vi "HyMPaCt Control Software.vi"() -> ()   [LabVIEW 2017]
doc: "This is the vi discription of the Top Level VI"
uses:
  LV Source/[meerstetter engineering TE Cooling]/TypeDefs/meTEC_ID 50000_Live Enable.ctl
  LV Source/[meerstetter engineering TE Cooling]/TypeDefs/meTEC_ID 2000_Input Selection.ctl
  LV Source/[meerstetter engineering TE Cooling]/TypeDefs/meTEC_ID 50011_Object Target Temperature Source Selection.ctl
  LV Source/[meerstetter engineering TE Cooling]/TypeDefs/meTEC_ID 104_Device Status.ctl
  LV Source/[meerstetter engineering TE Cooling]/TypeDefs/meTEC_ID 1200_Temperature is Stable.ctl
  LV Source/[meerstetter engineering TE Cooling]/TypeDefs/meTEC_ID 2010_Status.ctl
  LV Source/[HyMPaCt]/tec_global_typedef.ctl
  LV Source/Type Definitions/Main Loop Queue Data.ctl
  LV Source/Type Definitions/Main Loop States.ctl
  <vilib>/Platform/TimedLoop/XDataNode/timing_clust.ctl
  <vilib>/Platform/TimedLoop/XDataNode/nitl_modes.ctl
  <vilib>/Platform/TimedLoop/XDataNode/wakeup.ctl
  LV Source/Variables/FGVs/Type Defs/FGV_Operations.ctl
  <vilib>/Utility/error.llb/DialogType.ctl
  LV Source/[HyMPaCt]/log_file_typedef.ctl
  LV Source/[HyMPaCt]/record_typedef.ctl
  LV Source/Variables/Globals/Global_Quit.vi
  LV Source/Variables/Globals/Global_Initialized.vi
  LV Source/Variables/Globals/Global_TEC Monitor Loop_Status.vi
  <vilib>/platform/TimedLoop/XDataNode/XDataNode.xnode
  <vilib>/Platform/TimedLoop/XDataNode/XDNodeRunTimeDep.lvlib
panel:
  in  "Help Button":bool
  out "Reference timestamp 2":timestamp=timestamp(3582724140 s since 1904-01-01)
  in  "Numeric Control":T1
  in  "extra":string
  out "Control Suite Status":string
  in  "Tab Control_General":T2(tab)
  in  "Duration (minutes)":i32=30 caption="Duration (min)" min=-273 max=1000 step=1
  in  "Planned Recordings":i32(listbox)
  out "ARD_Object Temperature [°C] 2":dbl caption="Object Temperature 2 [°C]" format="%.3f"
  out "ARD_ Object Temperature [°C] 1":dbl caption="Object Temperature 1 [°C]" format="%.3f"
  in  "Reconnect Tec":bool caption="Reconnect Arduino"
  in  "Reconnect Arduino":bool
  out "TEC_connected":bool
  out "meTEC_Device Type":string caption="Device Type"
  out "meTEC_CH1_Device Status":T3=1 caption="Device Status" items=["Initializing", "Ready", "Run", "Error", "Bootloader", "Reset in Progress"]
  out "meTEC_CH1_Temperature Stability":T4=1 caption="Temperature Stabilty" items=["Temperature regulation is not active", "Is not stable", "Is stable"]
  out "meTEC_CH1_Object Temperature [°C]":dbl caption="Object Temperature [°C]" format="%.3f"
  out "meTEC_CH1_Sink Temperature [°C]":dbl caption="Sink Temperature [°C]" format="%.3f"
  out "meTEC_CH1_Act. Output Voltage [V]":dbl caption="Act. Output Voltage [V]" format="%.3f"
  out "meTEC_CH1_Act. Output Current [A]":dbl caption="Act. Output Current [A]" format="%.3f"
  out "meTEC_Hardware Version":string caption="Hardware Version"
  out "meTEC_Firmware Version":string caption="Firmware Version"
  out "meTEC_Serial No.":i32 caption="Serial No."
  out "meTEC_CH1_Error No.":i32 caption="Error No."
  out "meTEC_CH1_Error Instance":i32 caption="Error Instance"
  out "meTEC_CH1_Error Parameter":i32 caption="Error Parameter"
  out "TEC Log File":path=path "C:/Users/fedce/Desktop/prova101.xlsx"
  in  "meTEC_Reset Device 2":bool caption="Reset Device"
  out "Arduino Serial In":string
  in  "COM Port":refnum<visa-resource-name>="COM5"
  out "Arduino Connected":bool
  out "Reference timestamp":timestamp=timestamp(3582724140 s since 1904-01-01)
  in  "save log file":bool caption="Save Log Files"
  in  "Recording start time":timestamp=timestamp(3583143971.2784286 s since 1904-01-01) format="%<%H:%M %x>T"
  in  "Add recording":bool
  in  "meTEC_CH1_Status (ID 2010)":T5=2 caption="Status" items=["Static OFF", "Static ON", "Live OFF/ON", "HW Enable"]
  in  "meTEC_Reset Device":bool caption="Reset Device"
  in  "meTEC_CH1_Live Enable (ID 50000)":T6 caption="Live Enable (ID 50000)" items=["Disabled (Reset State)", "Enabled"]
  in  "meTEC_CH1_Input Selection (ID 2000)":T7=2 caption="Input  Selection (ID 2000)" items=["Static Current / Voltage", "Live Current / Voltage", "Temperature Controller"]
  in  "meTEC_CH1_Object Target Temp. Source Selection (ID 50011)":T8 caption="Object Target Temperature Source Selection (ID 50011)" items=["Parameter ID 3000 (Reset State)", "Parameter ID 50012"]
  in  "meTEC_CH1_Object Target Temperature (ID 3000 / 50012) [°C]":dbl=23.0 caption="Object Target Temperature (ID 3000 / 50012) [°C]" min=-273.0 max=1000.0 step=0.001 format="%#.3f"
  in  "meTEC_CH1_Live Set Current (ID 50001) [A]":dbl caption="Live Set Current (ID 50001) [A]" min=-16.0 max=16.0 step=0.001 format="%#.3f"
  in  "meTEC_CH1_Live Set Voltage (ID 50002) [V]":dbl caption="Live Set Voltage (ID 50002) [V]" min=0.0 max=30.0 step=0.001 format="%#.3f"
  in  "meTEC_Initialize Device":bool caption="Initialize Device"
  in  "Read Arduino Serial":bool caption="Initialize Device"
  out "Monitor Chart_CH1_Sink Temperature [°C]":dbl[](graph)
  out "Monitor Chart_CH1":dbl[](graph)
  out "Loop Rate [ms]":u32 caption="Update Rate [ms]"
  out "Monitor Chart_Current [A]":dbl[](graph)
  out "Monitor Chart_Voltage [V]":dbl[](graph)
  out "Loop Rate [ms] 2":u32 caption="Update Rate [ms]"
  out "Monitor Chart_ARD 2":i64(graph)
  out "Monitor Chart_ARD 1":i64(graph)
  in  "meTEC_Perform Test":bool caption="Execute Test"
  out "Error History Table":string[][](table) caption="Error History"
  in  "Filepath Error Log File":path=path "C:/Error Data"
  in  "Show Pop-Ups for Error Messages?":bool
  in  "meTEC_Error Test 1_ID100_Device Type":bool caption="Error Test"
  # "TEC General"
  # "TEC Data"
  # "Recording Options"
  # "Arduino Data"
  # "Channel 1"
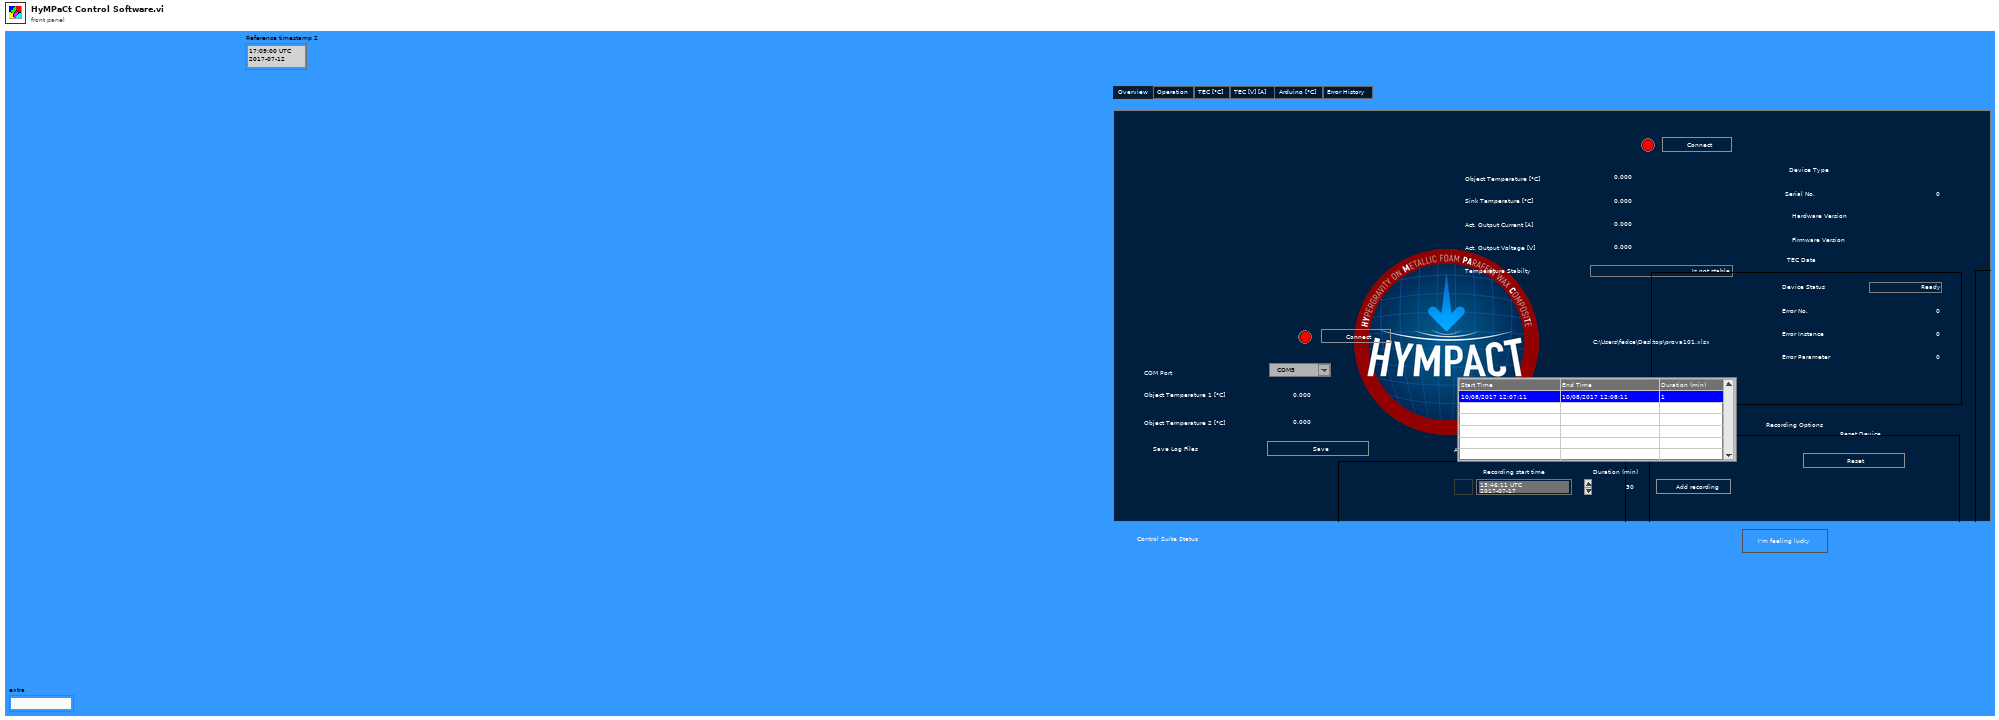
[diagram p1: front panel]
types:
  T1 = typedef "tec_global_typedef.ctl" = cluster{"Time Stamp":timestamp, "Voltage":dbl, "Current":dbl, "SinkT":dbl, "ObjT":dbl}
  T2 = enum32{"Overview", "Operation", "TEC [°C]", "TEC [V] [A]", "Arduino [°C]", "Error History"}
  T3 = typedef "meTEC_ID 104_Device Status.ctl" = i32
  T4 = typedef "meTEC_ID 1200_Temperature is Stable.ctl" = i32
  T5 = typedef "meTEC_ID 2010_Status.ctl" = i32
  T6 = typedef "meTEC_ID 50000_Live Enable.ctl" = i32
  T7 = typedef "meTEC_ID 2000_Input Selection.ctl" = i32
  T8 = typedef "meTEC_ID 50011_Object Target Temperature Source Selection.ctl" = i32
  T9 = typedef "Main Loop States.ctl" = enum16{"  -----  Core  -----  ", "Blank", "Idle", "Initialize", "Initialize Arduino", "Shutdown", "Error", "  ----- meerstetter TEC Functions -----  ", "TE Controller", " ----- Arduino Functions ----- ", "Read Arduino Serial", "Disconnect Arduino", "  -----  File manager  ----- ", "Start new recording", "Add recording", "Update table", "Save to log file"}
  T10 = typedef "Main Loop Queue Data.ctl" = cluster{"Parameter":string, "Variant":variant, "Main Loop States":T9}
  T11 = enum32{"invalid app kind", "Development System", "Run Time System", "Student Edition", "Embedded LabVIEW", "Evaluation", "Custom"}
  T12 = typedef "FGV_Operations.ctl" = enum16{"Read", "Read and delete", "Write"}
  T13 = typedef "FGV_TE Controller.ctl" = cluster{"SVs":cluster{"Unused":dbl}, "PVs":cluster{"FW & HW Versions":cluster{"Device Type [I32]":i32, "Device Type [String]":string, "Firmware Version [I32]":i32, "Firmware Version [String]":string, "Hardware Version [I32]":i32, "Hardware Version [String]":string, "Serial No.":i32}, "TEC Configuration":T14, "Object Target Temperature Source_CH1":u8, "Object Target Temperature Source_CH2":u8}, "Front Panel References":cluster{"Main Loop Queue":refnum<queue>, "meTEC_Device Type":refnum<vi>, "meTEC_Serial No.":refnum<vi>, "meTEC_Hardware Version":refnum<vi>, "meTEC_Firmware Version":refnum<vi>, "meTEC_CH1_Object Target Temperature (ID 3000 / 50012) [°C]":refnum<vi>, "meTEC_CH1_Live Set Current (ID 50001) [A]":refnum<vi>, "meTEC_CH1_Live Set Voltage (ID 50002) [V]":refnum<vi>, "meTEC_CH1_Live Enable (ID 50000)":refnum<vi>, "meTEC_CH1_Input Selection (ID 2000)":refnum<vi>, "meTEC_CH1_Object Target Temp. Source Sel. (ID 50011)":refnum<vi>, "meTEC_Initialize Device":refnum<vi>}, "TEC Log File":path, "Arduino VISA":refnum<visa-resource-name>}
  T14 = typedef "meTEC_Configuration.ctl" = cluster{"VISA resource name":refnum<visa-resource-name>, "Device Address":u16}
  T15 = typedef "XDNodeRunTimeDep.lvlib/timing_clust.ctl" = cluster{"Expected End [f-1]":u64, "Actual End [f-1]":u64, "Finished Late? [f-1]":bool, "Expected End [i-1]":u64, "Actual End [i-1]":u64, "Finished Late? [i-1]":bool, "Expected Start [i]":u64, "Actual Start [i]":u64, "Expected Start [f]":u64, "Actual Start [f]":u64, "Source Name":string, "Structure Name":string, "Period":i64, "Deadline":i64, "Offset":i64, "Start":i64, "Priority":i32, "Timeout":i32, "Mode":T16, "Wakeup Reason":T17, "Error":errorcluster, "Source Type":string, "Secondary Source Type":string, "Global End Time":u64, "Global Start Time":u64, "Frame Duration":u64, "Iteration Duration":u64, "Assigned CPU":i32, "I/O Scan Engine Mode":u32}
  T16 = typedef "XDNodeRunTimeDep.lvlib/nitl_modes.ctl" = enum32{"No Change", "Process missed periods, maintain original phase", "Discard missed periods, maintain original phase", "Process missed periods, ignore original phase", "Discard missed periods, ignore original phase"}
  T17 = typedef "XDNodeRunTimeDep.lvlib/wakeup.ctl" = enum32{"Normal", "Aborted", "Asynchronous wakeup", "Timing source error", "Timed loop error", "Timeout"}
  T18 = typedef "DialogType.ctl" = u16
  T19 = typedef "log_file_typedef.ctl" = cluster{"Type":string, "Sequence":u16, "Data":i64[], "CS":u16, "CRC":u16, "Time Stamp":timestamp, "Voltage":dbl, "Current":dbl, "TEC T_1":dbl, "TEC T_2":dbl}
  T20 = typedef "record_typedef.ctl" = cluster{"Start":timestamp, "Finish":timestamp, "Duration":i32}
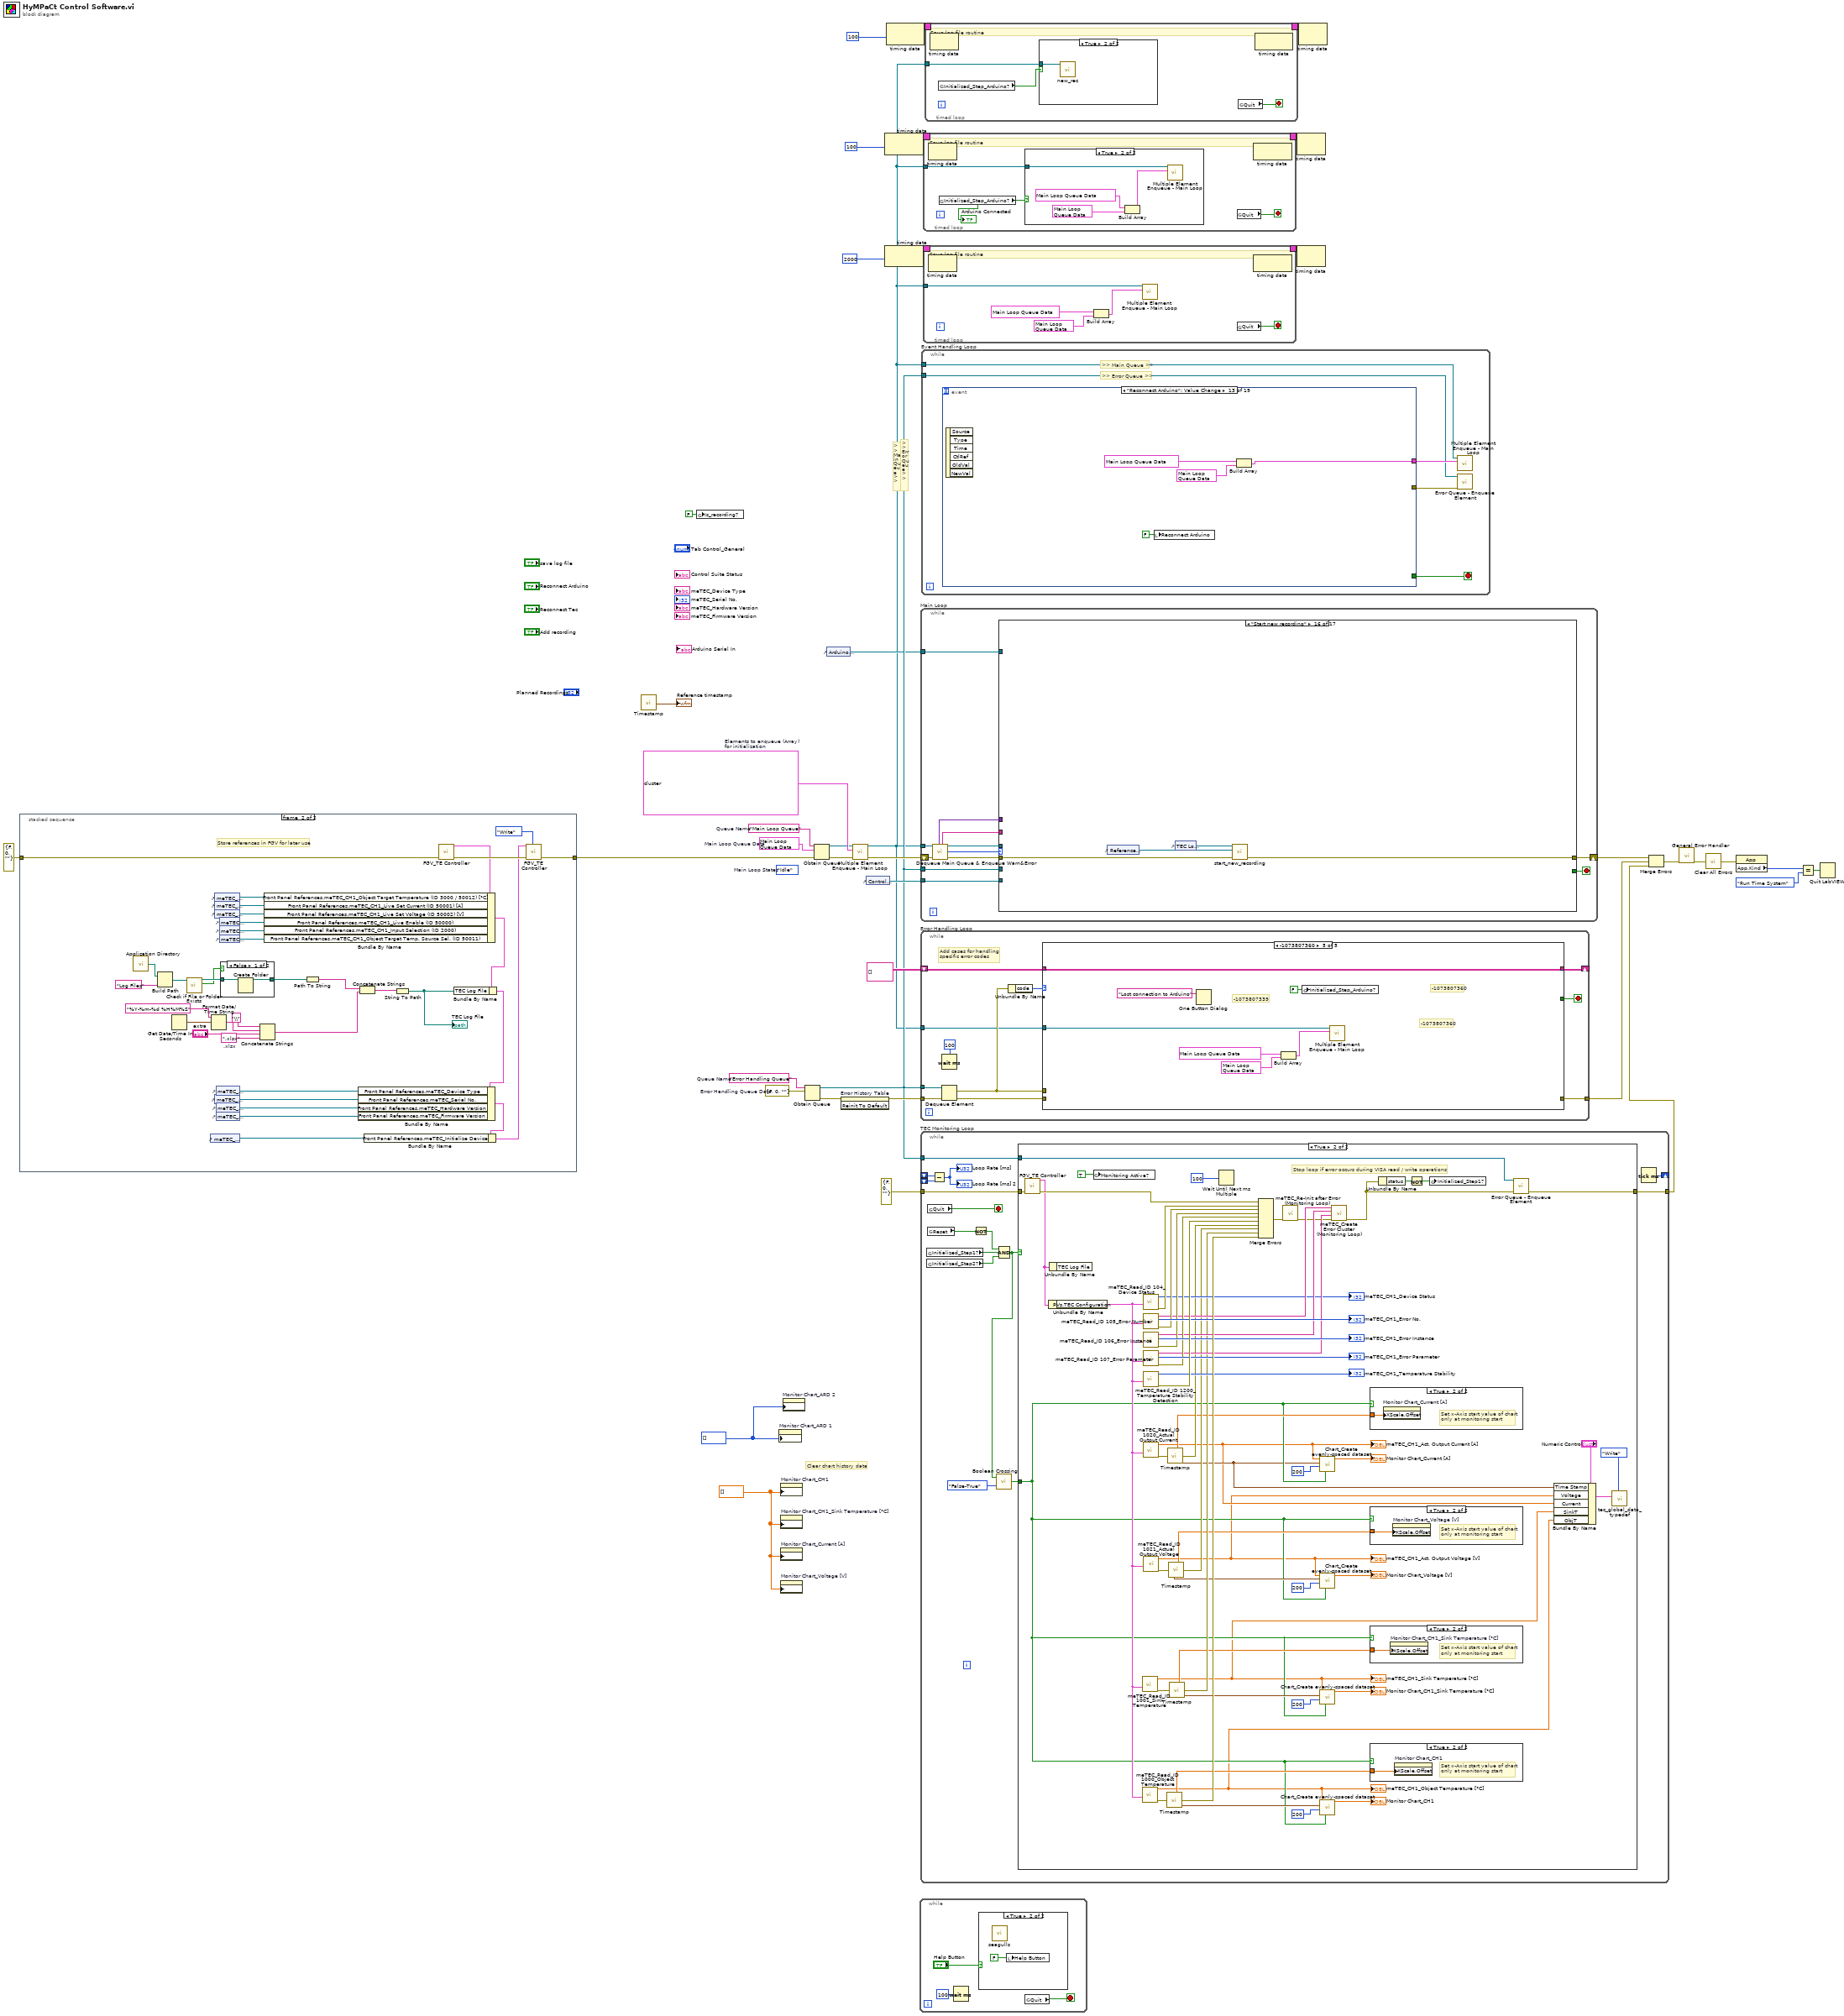
[diagram p0: block diagram]
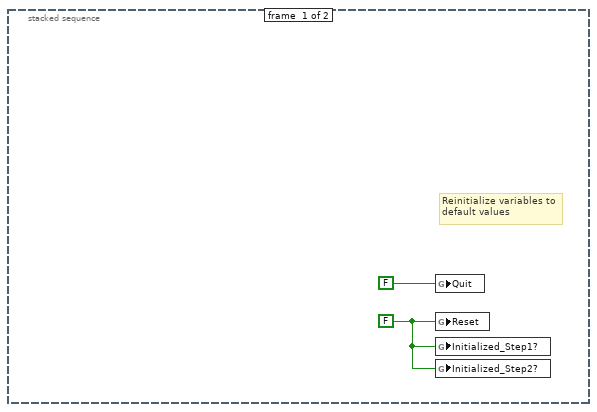
[diagram p5: hidden frame]
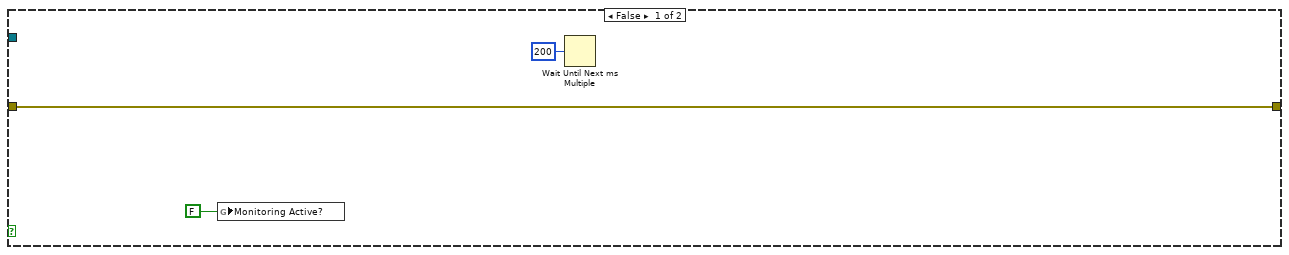
[diagram p7: hidden frame]
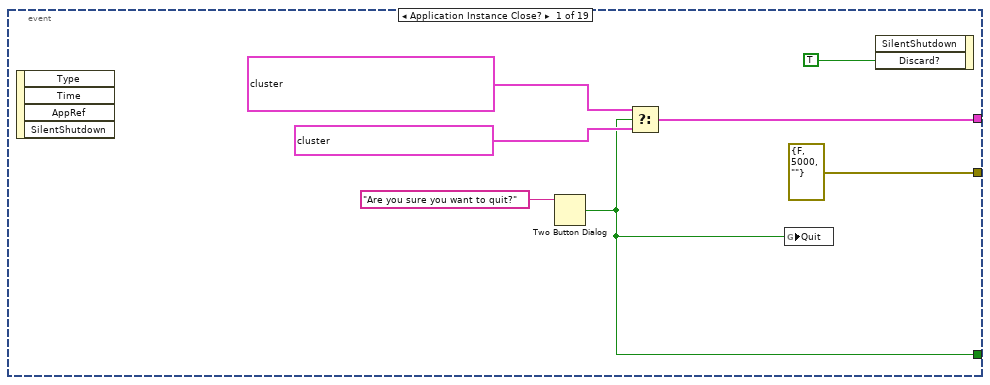
[diagram p12: hidden frame]
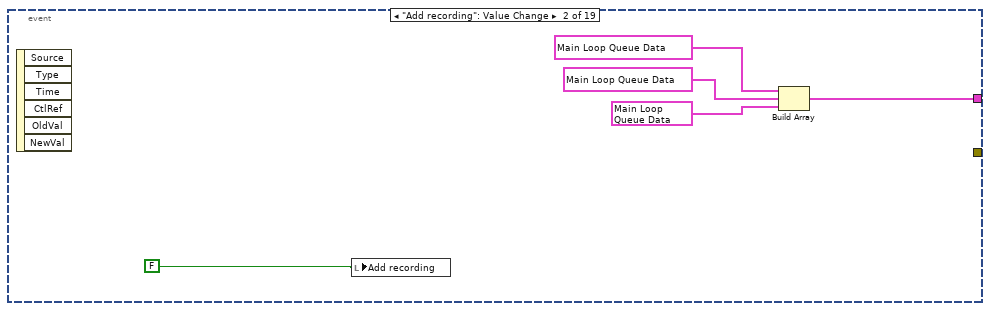
[diagram p13: hidden frame]
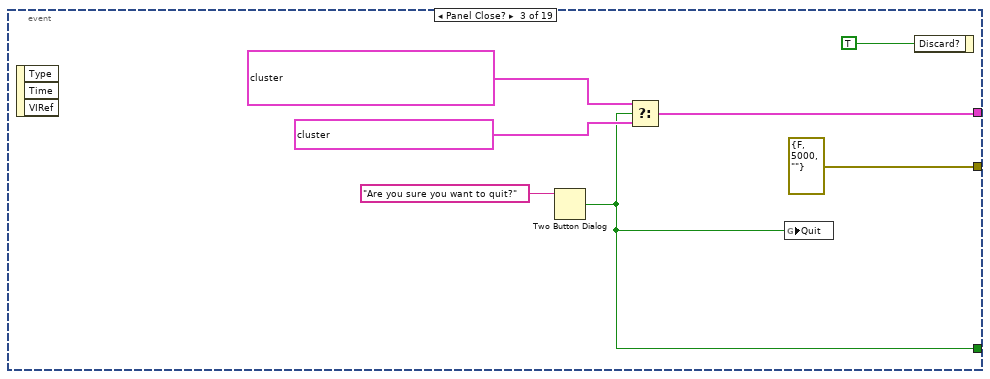
[diagram p14: hidden frame]
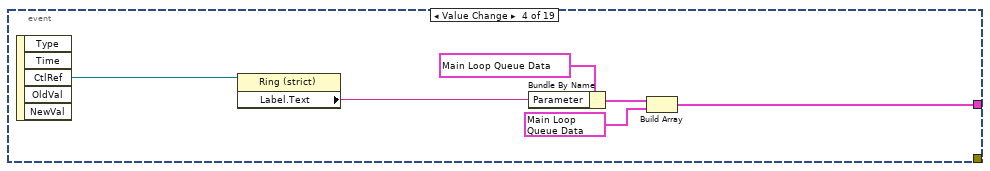
[diagram p15: hidden frame]
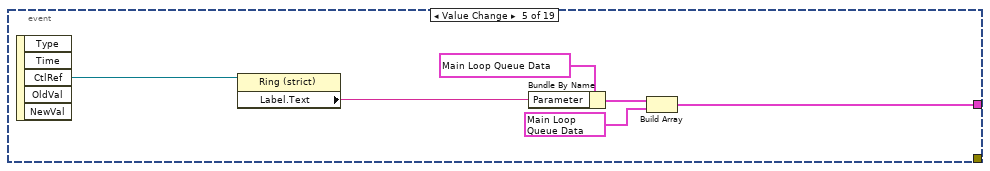
[diagram p16: hidden frame]
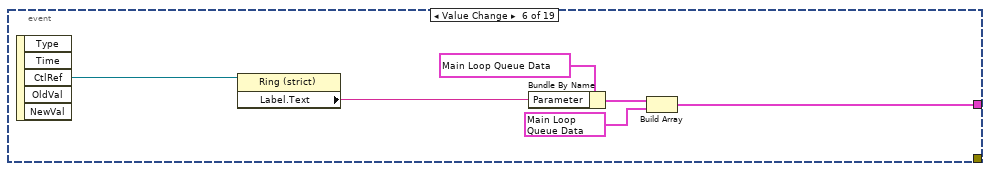
[diagram p17: hidden frame]
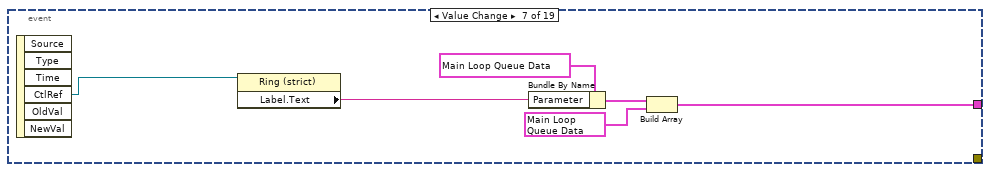
[diagram p18: hidden frame]
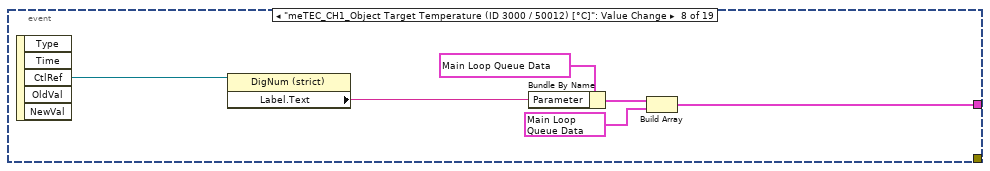
[diagram p19: hidden frame]
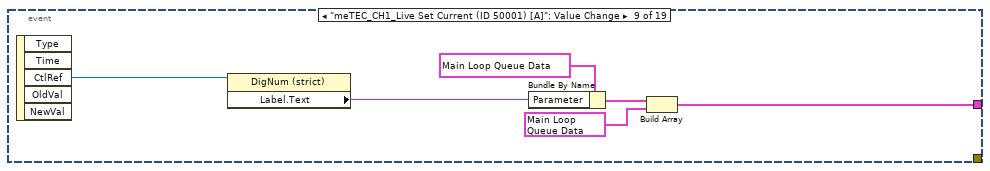
[diagram p20: hidden frame]
diagram:
  w14 = i64[] [] ("History Data")
  w18 = dbl[] [] ("History Data")
  (unwired) Main_Loop_States."Idle"  # Main Loop States
  w31 = T10 {"Parameter"="", "Variant"=variant, "Main Loop States"=enum."Idle"}  # Main Loop Queue Data
  w35 = errorcluster {"status"=FALSE, "code"=0, "source"=""}  # Error Handling Queue Data
  w36 = "Error Handling Queue"  # Queue Name
  w37 = "Main Loop Queue"  # Queue Name
  w30 = T10[] [{"Parameter"="", "Variant"=variant, "Main Loop States"=enum."Initialize"}, {"Parameter"="", "Variant"=variant, "Main Loop States"=enum."Initialize Arduino"}, {"Parameter"="", "Variant"=variant, "Main Loop States"=enum."Idle"}, {"Parameter"="", "Variant"=variant, "Main Loop States"=enum."Update table"}]  # Elements to enqueue (Array) for initialization
  # "Clear chart history data"
  # ">> Error Queue >>"
  # ">> Main Queue >>"
  n1 = stacked-sequence {
    tunnel: [_ w77] -> w24
    tunnel: errorcluster {"status"=FALSE, "code"=0, "source"=""} ("error out") -> [_ w78]
    frame #0 {
      w42 = FALSE ("Error")
      # "Reinitialize variables to\ndefault values"
      n2 = global write "Global_Quit.vi" "Quit"(FALSE ("Quit")) -> ()
      n3 = global write "Global_TEC Monitor Loop_Status.vi" "Reset"(w42) -> ()
      n4 = global write "Global_Initialized.vi" "Initialized_Step1?"(w42) -> ()
      n5 = global write "Global_Initialized.vi" "Initialized_Step2?"(w42) -> ()
    }
    frame #1 {
      w54 = ".xlsx"  # .xlsx
      # "Store references in FGV for later use"
      n6 = call <vilib>:"Application Directory.vi"() -> ("Application Directory"=w47:path)
      n7 = Build Path(base path=w47, name or relative path="Log Files" ("Folder")) -> (appended path=w46:path)
      n8 = Get Date/Time In Seconds() -> (seconds since 1Jan1904=w58:timestamp)
      n9 = call <vilib>:"Check if File or Folder Exists.vi"("path"=w46) -> ("file or folder exists?"=w44:bool, "dup path"=w45:path)  [unwired: 8 in, 1 out]
      n10 = control-ref of="meTEC_Initialize Device"() -> (w67:refnum<vi>)
      n11 = Format Date/Time String(time format string (%c)="%Y-%m-%d %H%M%S", seconds (now)=w58) -> (date/time string=w57:string)  [unwired: 1 in]
      n12 = control-ref of="meTEC_CH1_Object Target Temperature (ID 3000 / 50012) [°C]"() -> (w73:refnum<vi>)
      n13 = control-ref of="meTEC_CH1_Live Set Current (ID 50001) [A]"() -> (w71:refnum<vi>)
      n14 = control-ref of="meTEC_CH1_Live Set Voltage (ID 50002) [V]"() -> (w72:refnum<vi>)
      n15 = control-ref of="meTEC_Serial No."() -> (w64:refnum<vi>)
      n16 = control-ref of="meTEC_Device Type"() -> (w65:refnum<vi>)
      n17 = control-ref of="meTEC_Hardware Version"() -> (w63:refnum<vi>)
      n18 = control-ref of="meTEC_Firmware Version"() -> (w62:refnum<vi>)
      n19 = control-ref of="meTEC_CH1_Live Enable (ID 50000)"() -> (w61:refnum<vi>)
      n20 = control-ref of="meTEC_CH1_Input Selection (ID 2000)"() -> (w69:refnum<vi>)
      n21 = control-ref of="meTEC_CH1_Object Target Temp. Source Selection (ID 50011)"() -> (w68:refnum<vi>)
      n22 = case shown="False" w44 {
        tunnel: w45 -> [w80 w81]
        tunnel: [w79 w81] -> w43
        frame False {
          n23 = Create Folder(path (use dialog)=w80) -> (created path=w79:path)  [unwired: 2 in, 2 out]
        }
        frame True {
        }
      }
      n24 = Concatenate Strings("\\" ("string"), w57, "extra", w54) -> (w50:string)
      n25 = Path To String(path=w43) -> (string=w52:string)
      n26 = Concatenate Strings(w52, w50) -> (w51:string)
      n27 = String To Path(string=w51) -> (path=w49:path)
      "TEC Log File" <- w49
      n28 = call "FGV_TE Controller.vi"("error in (no error)"=w78) -> ("error out"=w76:errorcluster, "FGV_TEC_OUT"=w74:T13)  [unwired: 9 in]
      n29 = Bundle By Name(cluster=w74, "Front Panel References.meTEC_CH1_Object Target Temperature (ID 3000 / 50012) [°C]"=w73, "Front Panel References.meTEC_CH1_Live Set Current (ID 50001) [A]"=w71, "Front Panel References.meTEC_CH1_Live Set Voltage (ID 50002) [V]"=w72, "Front Panel References.meTEC_CH1_Live Enable (ID 50000)"=w61, "Front Panel References.meTEC_CH1_Input Selection (ID 2000)"=w69, "Front Panel References.meTEC_CH1_Object Target Temp. Source Sel. (ID 50011)"=w68) -> (w60:T13)
      n30 = Bundle By Name(cluster=w60, "TEC Log File"=w49) -> (w59:T13)
      n31 = Bundle By Name(cluster=w59, "Front Panel References.meTEC_Device Type"=w65, "Front Panel References.meTEC_Serial No."=w64, "Front Panel References.meTEC_Hardware Version"=w63, "Front Panel References.meTEC_Firmware Version"=w62) -> (w66:T13)
      n32 = Bundle By Name(cluster=w66, "Front Panel References.meTEC_Initialize Device"=w67) -> (w70:T13)
      n33 = call "FGV_TE Controller.vi"("Operation (Read)"=FGV_Operations."Write", "error in (no error)"=w76, "FGV_TEC_IN"=w70) -> ("error out"=w77:errorcluster)  [unwired: 7 in, 1 out]
    }
  }
  n34 = call "Timestamp.vi"() -> ("current time (time stamp)"=→"Reference timestamp":timestamp)  [unwired: 1 in, 2 out]
  n35 = global write "Global_Initialized.vi" "Is_recording?"(FALSE ("Is_recording?")) -> ()
  n36 = property on="Monitor Chart_ARD 1" class="WFChart (strict)"("History Data"=w14) -> ()  [unwired: 2 in, 2 out]
  n37 = property on="Monitor Chart_CH1" class="WFChart (strict)"("History Data"=w18) -> ()  [unwired: 2 in, 2 out]
  n38 = property on="Monitor Chart_CH1_Sink Temperature [°C]" class="WFChart (strict)"("History Data"=w18) -> ()  [unwired: 2 in, 2 out]
  n39 = property on="Monitor Chart_Current [A]" class="WFChart (strict)"("History Data"=w18) -> ()  [unwired: 2 in, 2 out]
  n40 = property on="Monitor Chart_Voltage [V]" class="WFChart (strict)"("History Data"=w18) -> ()  [unwired: 2 in, 2 out]
  n41 = property on="Monitor Chart_ARD 2" class="WFChart (strict)"("History Data"=w14) -> ()  [unwired: 2 in, 2 out]
  n42 = Obtain Queue(name (unnamed)=w36, element data type=w35) -> (queue out=w16:refnum<queue>, error out=w21:errorcluster)  [unwired: 3 in, 1 out]
  n43 = Obtain Queue(name (unnamed)=w37, element data type=w31, error in (no error)=w24) -> (queue out=w29:refnum<queue>, error out=w25:errorcluster)  [unwired: 2 in, 1 out]
  n44 = control-ref of="Arduino Serial In"() -> (w15:refnum<vi>)
  n45 = invoke on="Error History Table" class="Tbl (strict)" method="Reinit To Default"(error in=w21) -> (error out=w20:errorcluster)  [unwired: 2 in, 2 out]
  n46 = call "Multiple Element Enqueue - Main Loop.vi"("error in (no error)"=w25, "Elements to enqueue (Array)"=w30, "Queue In"=w29) -> ("error out"=w19:errorcluster, "QueueOut"=w1:refnum<queue>)  [unwired: 7 in]
  n47 = control-ref of="Control Suite Status"() -> (w27:refnum<vi>)
  n48 = node-c288(u32 100 ("millisecond multiple")) -> (w7:T15)
  n49 = node-c288(u32 2000 ("millisecond multiple")) -> (w11:T15)
  n50 = node-c288(u32 100 ("millisecond multiple")) -> (w4:T15)
  n51 = while {
    stop <- w82 stop-if-true
    n52 = Wait (ms)(milliseconds to wait=u32 100) -> ()  [unwired: 1 out]
    n53 = case shown="True" "Help Button" {
      frame False {
      }
      frame True {
        n54 = call "seagulls.vi"() -> ()  [unwired: 12 in]
        n55 = local write "Help Button"(FALSE ("Open Preheating")) -> ()
      }
    }
    n56 = global read "Global_Quit.vi" "Quit"() -> (w82:bool)
  }
  n57 = while "Error Handling Loop" {
    tunnel: w16 -> [w96]
    shift-right: [w91] -> _
    shift-left: string[][] [] -> [w90]
    tunnel: w20 -> [w95]
    tunnel: [w94] -> w34
    tunnel: w1 -> [w86]
    stop <- w92 stop-if-true
    # "Add cases for handling\nspecific error codes"
    n58 = Wait (ms)(milliseconds to wait=u32 100) -> ()  [unwired: 1 out]
    n59 = Dequeue Element(queue=w96, error in (no error)=w95) -> (element=w88:errorcluster, error out=w87:errorcluster)  [unwired: 1 in, 2 out]
    n60 = Unbundle By Name(w88) -> ("code"=w89:i32)
    n61 = case shown="-1073807360" w89 {
      tunnel: [_ _ w121 _ _] -> w94
      tunnel: w88 -> [w103 _ _ _ _]
      tunnel: [_ _ TRUE _ _] -> w92
      tunnel: [w110 w120 w123 w124 w129] -> w91
      tunnel: w90 -> [w109 w120 w123 w124 w129]
      tunnel: w87 -> [w106 _ w121 _ _]
      tunnel: w86 -> [_ _ _ _ w125]
      frame 1, Default {
        n62 = call "Error_Log to File.vi"("Error Log Filepath"="Filepath Error Log File", "error in (no error)"=w106, "Error Data_IN"=w103, "Error Log Filename"="ErrorLog.txt" ("Rel. Path\\Filename")) -> ("error out"=w108:errorcluster, "Error Data_OUT"=w102:errorcluster, "Error Data (2D String Array)"=w99:string[][], "Call chain empty?"=w97:bool)  [unwired: 4 in]
        n63 = Index Array(array=w99, index (row) #1=0 ("index (row)")) -> (element #1=w100:string[], element #2=w98:string[])  [unwired: 3 in]
        n64 = case shown="True" "Show Pop-Ups for Error Messages?" {
          tunnel: w102 -> [_ w119]
          frame False {
          }
          frame True {
            w118 = T18 3 items=["no dialog", "OK message", "continue or stop message", "OK message + warnings", "continue/stop + warnings"] ("type of dialog (OK msg:1)")
            n65 = call <vilib>:"General Error Handler.vi"("type of dialog (OK msg:1)"=w118, "error in (no error)"=w119) -> ()  [unwired: 9 in, 5 out]
          }
        }
        n66 = case shown="False" w97 {
          tunnel: [w114 w117] -> w110
          tunnel: w109 -> [w113 w116]
          tunnel: w100 -> [w112 w115]
          tunnel: w98 -> [w111 _]
          frame False {
            n67 = Build Array (concatenate)(w112, w111, w113) -> (w114:string[][])
          }
          frame True {
            n68 = Build Array (concatenate)(w115, w116) -> (w117:string[][])
          }
        }
        "Error History Table" <- w110
        n69 = call <vilib>:"Simple Error Handler.vi"("error in (no error)"=w108) -> ()  [unwired: 4 in, 5 out]
      }
      frame 1073676294 {
        # "Don't really care"
      }
      frame 5000 {
        # "Application quit by user request"
      }
      frame 501000, 502000 {
        # "These error codes to not correspond to any\ncommunication or device errors but represent\noffsets used to shift meerstetter engineering error\ncodes & numbers to LabVIEW user-specified error code ranges.\n\n-> see LabVIEW help and explanations in:\n1) meTEC_Create Error Cluster.vi\n2) meTEC_Check for Communication Error.vi\n3) meTEC_Check for Device Error.vi"
      }
      frame -1073807360 {
        # "-1073807339"
        # "-1073807360"
        # "-1073807360"
        n70 = One Button Dialog(message="Lost connection to Arduino") -> ()  [unwired: 1 in, 1 out]
        n71 = Build Array(T10 {"Parameter"="", "Variant"=variant, "Main Loop States"=enum."Disconnect Arduino"} ("Main Loop Queue Data"), T10 {"Parameter"="", "Variant"=variant, "Main Loop States"=enum."Idle"} ("Main Loop Queue Data")) -> (w126:T10[])
        n72 = global write "Global_Initialized.vi" "Initialized_Step_Arduino?"(FALSE ("Initialized_Step_Arduino?")) -> ()
        n73 = call "Multiple Element Enqueue - Main Loop.vi"("Elements to enqueue (Array)"=w126, "Queue In"=w125) -> ()  [unwired: 8 in, 2 out]
      }
    }
  }
  n74 = while "TEC Monitoring Loop" {
    tunnel: errorcluster {"status"=FALSE, "code"=0, "source"=""} ("error in") -> [w145]
    tunnel: w16 -> [w146]
    tunnel: [w144] -> w17
    shift-right: [w143] -> _
    shift-left: _ -> [w142]
    shift-left: _ -> [w141]
    stop <- w134 stop-if-true
    n75 = global read "Global_Initialized.vi" "Initialized_Step1?"() -> (w137:bool)
    n76 = global read "Global_Initialized.vi" "Initialized_Step2?"() -> (w138:bool)
    n77 = global read "Global_Quit.vi" "Quit"() -> (w134:bool)
    n78 = global read "Global_TEC Monitor Loop_Status.vi" "Reset"() -> (w140:bool)
    n79 = Subtract(x=w142, y=w141) -> (x-y=→"Loop Rate [ms]" →"Loop Rate [ms] 2":u32)
    n80 = Not(x=w140) -> (.not. x?=w139:bool)
    n81 = Compound Arithmetic op=AND(w139, w137, w138) -> (w136:bool)
    n82 = call "Boolean Crossing.vi"("Direction"=enum8{"Either", "False-True", "True-False"}."False-True", "Input"=w136) -> ("Crossing"=w135:bool)  [unwired: 1 in]
    n83 = case shown="True" w136 {
      tunnel: w145 -> [w149 w204]
      tunnel: [w149 w206] -> w144
      tunnel: w146 -> [_ w207]
      tunnel: w135 -> [_ w159]
      frame False {
        n84 = global write "Global_TEC Monitor Loop_Status.vi" "Monitoring Active?"(FALSE ("Error")) -> ()
        n85 = Wait Until Next ms Multiple(millisecond multiple=u32 200) -> ()  [unwired: 1 out]
      }
      frame True {
        # "Stop loop if error occurs during VISA read / write operations"
        n86 = call "FGV_TE Controller.vi"("error in (no error)"=w204) -> ("error out"=w203:errorcluster, "FGV_TEC_OUT"=w158:T13)  [unwired: 9 in]
        n87 = Unbundle By Name(w158) -> ("PVs.TEC Configuration"=w191:T14)
        n88 = Unbundle By Name(w158) -> ()  [unwired: 1 out]
        n89 = global write "Global_TEC Monitor Loop_Status.vi" "Monitoring Active?"(TRUE ("Error")) -> ()
        n90 = call "meTEC_Read_ID 1001_Sink Temperature.vi"("TEC Configuration_IN"=w191) -> ("error out"=w176:errorcluster, "Sink Temperature [°C] (ID 1001)"=w151:dbl)  [unwired: 8 in, 1 out]
        "meTEC_CH1_Sink Temperature [°C]" <- w151
        n91 = call "meTEC_Read_ID 1000_Object Temperature.vi"("TEC Configuration_IN"=w191) -> ("error out"=w201:errorcluster, "Object Temperature [°C] (ID 1000)"=w150:dbl)  [unwired: 8 in, 1 out]
        "meTEC_CH1_Object Temperature [°C]" <- w150
        n92 = call "meTEC_Read_ID 104_Device Status.vi"("TEC Configuration_IN"=w191) -> ("error out"=w198:errorcluster, "Device Status (ID 104) [I32]"=→"meTEC_CH1_Device Status":i32)  [unwired: 8 in, 1 out]
        n93 = call "meTEC_Read_ID 105_Error Number.vi"("TEC Configuration_IN"=w191) -> ("error out"=w194:errorcluster, "Error Number (ID 105) [I32]"=→"meTEC_CH1_Error No.":i32, "Error Number (ID 105) [String]"=w183:string)  [unwired: 7 in, 1 out]
        n94 = call "meTEC_Read_ID 106_Error Instance.vi"("TEC Configuration_IN"=w191) -> ("error out"=w193:errorcluster, "Error Instance (ID 106) [I32]"=→"meTEC_CH1_Error Instance":i32, "Error Instance (ID 106) [String]"=w184:string)  [unwired: 7 in, 1 out]
        n95 = call "meTEC_Read_ID 107_Error Parameter.vi"("TEC Configuration_IN"=w191) -> ("error out"=w192:errorcluster, "Error Parameter (ID 107) [I32]"=→"meTEC_CH1_Error Parameter":i32, "Error Parameter (ID 107) [String]"=w185:string)  [unwired: 7 in, 1 out]
        n96 = call "meTEC_Read_ID 1200_Temperature Stability Detection.vi"("TEC Configuration_IN"=w191) -> ("error out"=w202:errorcluster, "Temperature is Stable? [I32)] (ID 1200)"=→"meTEC_CH1_Temperature Stability":i32)  [unwired: 7 in, 2 out]
        n97 = call "meTEC_Read_ID 1020_Actual Output Current.vi"("TEC Configuration_IN"=w191) -> ("error out"=w168:errorcluster, "Act. Output Current [A] (ID 1020)"=w153:dbl)  [unwired: 8 in, 1 out]
        "meTEC_CH1_Act. Output Current [A]" <- w153
        n98 = call "meTEC_Read_ID 1021_Actual Output Voltage.vi"("TEC Configuration_IN"=w191) -> ("error out"=w174:errorcluster, "Act. Output Voltage [A] (ID 1021)"=w152:dbl)  [unwired: 8 in, 1 out]
        "meTEC_CH1_Act. Output Voltage [V]" <- w152
        n99 = call "Timestamp.vi"("error in (no error)"=w201) -> ("current time (time stamp)"=w160:timestamp, "current time (sec)"=w161:dbl, "error out"=w200:errorcluster)
        n100 = call "Timestamp.vi"("error in (no error)"=w168) -> ("current time (time stamp)"=w154:timestamp, "current time (sec)"=w164:dbl, "error out"=w167:errorcluster)
        n101 = call "Timestamp.vi"("error in (no error)"=w174) -> ("current time (time stamp)"=w171:timestamp, "current time (sec)"=w169:dbl, "error out"=w173:errorcluster)
        n102 = call "Timestamp.vi"("error in (no error)"=w176) -> ("current time (time stamp)"=w162:timestamp, "current time (sec)"=w163:dbl, "error out"=w175:errorcluster)
        n103 = Wait Until Next ms Multiple(millisecond multiple=u32 100 ("TEC_Loop wait time [ms]")) -> ()  [unwired: 1 out]
        n104 = Merge Errors(w203, w198, w194, w193, w192, w202, w167, w173, w175, w200) -> (w187:errorcluster)
        n105 = call "meTEC_Re-Init after Error (Monitoring Loop).vi"("error in (no error)"=w187) -> ("error out"=w180:errorcluster)  [unwired: 10 in]
        n106 = call "Chart_Create evenly-spaced dataset.vi"("Initialize?"=w159, "X-Axis Time Interval (100) [ms]"=200, "X (Time Stamp)"=w154, "Y (DBL)"=w153) -> ("Y (Interpolated array)"=→"Monitor Chart_Current [A]":dbl[])  [unwired: 6 in, 1 out]
        n107 = call "Chart_Create evenly-spaced dataset.vi"("Initialize?"=w159, "X-Axis Time Interval (100) [ms]"=200, "X (Time Stamp)"=w171, "Y (DBL)"=w152) -> ("Y (Interpolated array)"=→"Monitor Chart_Voltage [V]":dbl[])  [unwired: 6 in, 1 out]
        n108 = call "Chart_Create evenly-spaced dataset.vi"("Initialize?"=w159, "X-Axis Time Interval (100) [ms]"=200, "X (Time Stamp)"=w162, "Y (DBL)"=w151) -> ("Y (Interpolated array)"=→"Monitor Chart_CH1_Sink Temperature [°C]":dbl[])  [unwired: 6 in, 1 out]
        n109 = call "Chart_Create evenly-spaced dataset.vi"("Initialize?"=w159, "X-Axis Time Interval (100) [ms]"=200, "X (Time Stamp)"=w160, "Y (DBL)"=w150) -> ("Y (Interpolated array)"=→"Monitor Chart_CH1":dbl[])  [unwired: 6 in, 1 out]
        n110 = call "meTEC_Create Error Cluster (Monitoring Loop).vi"("error in (no error)"=w180, "Error Parameter"=w185, "Error Instance"=w184, "Error Number"=w183) -> ("error out"=w186:errorcluster)  [unwired: 7 in]
        n111 = case shown="True" w159 {
          tunnel: w164 -> [_ w208]
          frame False {
          }
          frame True {
            # "Set x-Axis start value of chart\nonly at monitoring start"
            n112 = property on="Monitor Chart_Current [A]" class="WFChart (strict)"("XScale.Offset"=w208) -> ()  [unwired: 2 in, 2 out]
          }
        }
        n113 = case shown="True" w159 {
          tunnel: w169 -> [_ w209]
          frame False {
          }
          frame True {
            # "Set x-Axis start value of chart\nonly at monitoring start"
            n114 = property on="Monitor Chart_Voltage [V]" class="WFChart (strict)"("XScale.Offset"=w209) -> ()  [unwired: 2 in, 2 out]
          }
        }
        n115 = case shown="True" w159 {
          tunnel: w163 -> [_ w210]
          frame False {
          }
          frame True {
            # "Set x-Axis start value of chart\nonly at monitoring start"
            n116 = property on="Monitor Chart_CH1_Sink Temperature [°C]" class="WFChart (strict)"("XScale.Offset"=w210) -> ()  [unwired: 2 in, 2 out]
          }
        }
        n117 = case shown="True" w159 {
          tunnel: w161 -> [_ w211]
          frame False {
          }
          frame True {
            # "Set x-Axis start value of chart\nonly at monitoring start"
            n118 = property on="Monitor Chart_CH1" class="WFChart (strict)"("XScale.Offset"=w211) -> ()  [unwired: 2 in, 2 out]
          }
        }
        n119 = Unbundle By Name(w186) -> ("status"=w182:bool)
        n120 = Not(x=w182) -> (.not. x?=w181:bool)
        n121 = global write "Global_Initialized.vi" "Initialized_Step1?"(w181) -> ()
        n122 = call "Error Queue - Enqueue Element.vi"("error in (no error)"=w186, "Error Queue IN"=w207) -> ("error out"=w206:errorcluster)  [unwired: 9 in]
        n123 = Bundle By Name(cluster="Numeric Control", "Time Stamp"=w154, "Voltage"=w152, "Current"=w153, "SinkT"=w151, "ObjT"=w150) -> (w156:T1)
        n124 = call "tec_global_data_typedef.vi"("Operation (Read)"=FGV_Operations."Write", "Numeric Control"=w156) -> ()  [unwired: 9 in, 1 out]
      }
    }
    n125 = Tick Count (ms)() -> (millisecond timer value=w143:u32)
  }
  n126 = while "Main Loop" {
    tunnel: w1 -> [w221]
    tunnel: w16 -> [w222]
    tunnel: w27 -> [w214]
    tunnel: w15 -> [w213]
    shift-right: [w212] -> w8
    shift-left: w19 -> [w220]
    stop <- w223 stop-if-true
    n127 = call "Dequeue Main Queue & Enqueue Warn&Error.vi"("error in (no error)"=w220, "Queue In"=w221) -> ("error out (no error)"=w219:errorcluster, "Main Loop State"=w217:T9, "Queue Out"=w218:refnum<queue>, "Parameter"=w216:string, "Variant"=w215:variant)  [unwired: 5 in]
    n128 = case shown="\"Start new recording\"" w217 {
      tunnel: [_ _ _ _ _ TRUE _ _ _ _ _ _ _ _ _ _ _] -> w223
      tunnel: w219 -> [_ _ _ w245 w254 w257 w269 _ w283 _ w413 _ _ _ _ w481 _]
      tunnel: w222 -> [_ _ _ w244 w253 w260 w270 _ _ _ _ _ _ _ _ _ _]
      tunnel: w218 -> [_ _ _ _ _ _ w267 _ w279 _ w414 _ _ _ _ _ _]
      tunnel: w216 -> [_ _ _ _ _ _ _ _ w281 _ _ _ _ _ _ _ _]
      tunnel: w215 -> [_ _ _ _ _ _ _ _ _ _ _ _ _ _ _ _ _]
      tunnel: w214 -> [_ w225 w227 w243 w252 w258 _ _ w282 _ _ _ _ _ _ _ _]
      tunnel: w213 -> [_ _ _ _ _ _ _ _ _ _ w412 _ _ _ _ _ _]
      tunnel: [_ _ _ w238 w249 w256 w261 _ w278 _ w410 _ _ _ _ w480 w482] -> w212
      frame "  -----  Core  -----  " {
      }
      frame "Blank" {
        n129 = property class="Str"(reference=w225, "Value"="Process Description...") -> ()  [unwired: 1 in, 2 out]
      }
      frame "Idle", Default {
        n130 = global read "Global_Initialized.vi" "Initialized_Step1?"() -> (w226:bool)
        "TEC_connected" <- w226
        n131 = case shown="False" w226 {
          tunnel: w227 -> [w229 w234]
          frame True {
            n132 = global read "Global_Initialized.vi" "Initialized_Step_Arduino?"() -> (w228:bool)
            n133 = Select(t="Idle" ("Value"), s=w228, f="TEC connected, no TE Arduino connected!" ("Value")) -> (s? t:f=w230:string)
            n134 = property class="Str"(reference=w229, "Value"=w230) -> ()  [unwired: 1 in, 2 out]
          }
          frame False {
            n135 = global read "Global_Initialized.vi" "Initialized_Step_Arduino?"() -> (w233:bool)
            n136 = Select(t="Arduino connected, no TEC connected!" ("Value"), s=w233, f="No TE Arduino connected, no Arduino connected!" ("Value")) -> (s? t:f=w235:string)
            n137 = property class="Str"(reference=w234, "Value"=w235) -> ()  [unwired: 1 in, 2 out]
          }
        }
      }
      frame "Initialize" {
        # "Initialize TE Controller"
        n138 = call "Initialize System.vi"("System Status"=w243, "Error Queue"=w244, "error in (no error)"=w245, "Array"=string[] ["Initialize TEC System", "Read TEC Characteristics", "Update Front Panel", "Configure Front Panel", "Finish Initialization", ""]) -> ("error out"=w241:errorcluster)  [unwired: 7 in]
        n139 = call "record_sessions.vi"("error in (no error)"=w241) -> ("error out"=w240:errorcluster, "record sessions"=w239:T20[])  [unwired: 9 in]
        n140 = for {
          tunnel: w239 -> [_] mode=indexing
          shift-right: [w246] -> w238
          shift-left: w240 -> [w248]
          n141 = call "record_sessions.vi"("Operation (Read)"=FGV_Operations."Read and delete", "error in (no error)"=w248) -> ("error out"=w246:errorcluster)  [unwired: 8 in, 1 out]
        }
      }
      frame "Initialize Arduino" {
        n142 = call "Initialize System.vi"("System Status"=w252, "Error Queue"=w253, "error in (no error)"=w254, "Array"=string[] ["Initialize Arduino", "Finish Initialization", "", "", "", ""], "COM Port"="COM Port") -> ("error out"=w249:errorcluster)  [unwired: 6 in]
        n143 = local write "save log file"(FALSE ("save log file")) -> ()
      }
      frame "Shutdown" {
        n144 = call "Shutdown System.vi"("System Status"=w258, "Error Queue"=w260, "error in (no error)"=w257) -> ("error out"=w256:errorcluster)  [unwired: 8 in]
      }
      frame "Error" {
        (unwired) i32[] []
        # "List all error codes in this array which require a queue flush"
        n145 = Unbundle By Name(w269) -> ("code"=w268:i32, "status"=w263:bool)
        n146 = Enqueue Element(queue=w270, element=w269) -> (error out=w266:errorcluster)  [unwired: 2 in, 2 out]
        n147 = Equal?(x=-8000, y=w268) -> (x = y?=w264:bool)
        n148 = And(x=w264, y=w263) -> (x .and. y?=w262:bool)
        n149 = case shown="True" w262 {
          tunnel: w267 -> [_ w277]
          tunnel: w266 -> [w271 w276]
          tunnel: [w271 w274] -> w261
          frame False {
          }
          frame True {
            # "Execute specified\nstates in case of error"
            # "Flush Queue"
            n150 = Flush Queue(queue=w277, error in (no error)=w276) -> (queue out=w273:refnum<queue>, error out=w275:errorcluster)  [unwired: 1 out]
            n151 = call "Multiple Element Enqueue - Main Loop.vi"("error in (no error)"=w275, "Elements to enqueue (Array)"=T10[] [], "Queue In"=w273) -> ("error out"=w274:errorcluster)  [unwired: 7 in, 1 out]
          }
        }
      }
      frame "  ----- meerstetter TEC Functions -----  " {
      }
      frame "TE Controller" {
        n152 = call "FGV_TE Controller.vi"() -> ("FGV_TEC_OUT"=w280:T13)  [unwired: 10 in, 1 out]
        n153 = case shown="\"meTEC_Perform Test\"" w281 {
          tunnel: w283 -> [w284 w298 w326 w334 w339 w352 w360 w369 w387 w395 w400 w406]
          tunnel: [w284 w296 w326 w333 w338 w351 w359 w368 w386 w394 w398 w404] -> w278
          tunnel: w282 -> [w286 w300 w328 w336 w344 w354 w362 w371 w389 w397 w403 w409]
          tunnel: w280 -> [_ w297 _ w332 w342 w348 w358 w366 w385 w393 w401 w407]
          tunnel: w279 -> [_ w290 _ _ _ _ _ _ _ _ _ _]
          frame "Blank", Default {
            n154 = property class="Str"(reference=w286, "Value"="To do...") -> ()  [unwired: 1 in, 2 out]
          }
          frame "meTEC_Reset Device" {
            n155 = flat-sequence {
              tunnel: w297 -> [w303]
              tunnel: w298 -> [w304]
              tunnel: [w304] -> w295
              tunnel: [w303] -> w294
              tunnel: w290 -> [w301]
              tunnel: [w301] -> w289
              tunnel: w295 -> [w312]
              tunnel: w294 -> [w311]
              tunnel: [w310] -> w293
              tunnel: [w309] -> w292
              tunnel: w289 -> [w307]
              tunnel: [w307] -> w287
              tunnel: w293 -> [w318]
              tunnel: w292 -> [w316]
              tunnel: [w317] -> w291
              tunnel: [w313] -> w288
              tunnel: w287 -> [w313]
              tunnel: [w321] -> w296
              tunnel: w291 -> [w322]
              tunnel: w288 -> [w320]
              frame #0 {
                # "Stop monitoring loop and wait\nuntil it actually stopped"
                n156 = while {
                  stop <- w306 continue-if-true
                  n157 = global read "Global_TEC Monitor Loop_Status.vi" "Monitoring Active?"() -> (w306:bool)
                  n158 = Wait Until Next ms Multiple(millisecond multiple=u32 50) -> ()  [unwired: 1 out]
                }
                n159 = global write "Global_TEC Monitor Loop_Status.vi" "Reset"(TRUE ("Reset")) -> ()
              }
              frame #1 {
                # "Reset TEC"
                n160 = Unbundle By Name(w311) -> ("PVs.TEC Configuration"=w309:T14)
                n161 = global write "Global_Initialized.vi" "Initialized_Step1?"(FALSE ("Initialized_Step1?")) -> ()
                n162 = call "meTEC_Reset Device.vi"("error in (no error)"=w312, "TEC Configuration_IN"=w309) -> ("error out"=w310:errorcluster)  [unwired: 7 in, 2 out]
              }
              frame #2 {
                # "Close COM port"
                n163 = Unbundle By Name(w316) -> ("VISA resource name"=w315:refnum<visa-resource-name>)
                n164 = Wait (ms)(milliseconds to wait=u32 200) -> ()  [unwired: 1 out]
                n165 = VISA Close(VISA resource name=w315, error in (no error)=w318) -> (error out=w317:errorcluster)
              }
              frame #3 {
                w319 = T10[] [{"Parameter"="", "Variant"=variant, "Main Loop States"=enum."Initialize"}, {"Parameter"="", "Variant"=variant, "Main Loop States"=enum."Idle"}]  # Elements to enqueue (Array) for initialization
                # "Trigger initialization\nprocess"
                n166 = global write "Global_TEC Monitor Loop_Status.vi" "Reset"(FALSE ("Reset")) -> ()
                n167 = call "Multiple Element Enqueue - Main Loop.vi"("error in (no error)"=w322, "Elements to enqueue (Array)"=w319, "Queue In"=w320) -> ("error out"=w321:errorcluster)  [unwired: 7 in, 1 out]
              }
            }
            n168 = property class="Str"(reference=w300, "Value"="Resetting TEC...") -> ()  [unwired: 1 in, 2 out]
          }
          frame "Return Front Panel Controls to TEC Reset State" {
            w324 = 0 items=["Parameter ID 3000 (Reset State)", "Parameter ID 50012"]
            w325 = 0 items=["Disabled (Reset State)", "Enabled"]
            n169 = property on="meTEC_CH1_Live Enable (ID 50000)" class="Ring (strict)"("Value"=w325) -> ()  [unwired: 2 in, 2 out]
            n170 = property on="meTEC_CH1_Object Target Temp. Source Selection (ID 50011)" class="Ring (strict)"("Value"=w324) -> ()  [unwired: 2 in, 2 out]
            n171 = property class="Str"(reference=w328, "Value"="Returning Front Panel Controls to TEC Reset State..") -> ()  [unwired: 1 in, 2 out]
          }
          frame "meTEC_CH1_Input Selection (ID 2000)" {
            n172 = Unbundle By Name(w332) -> ("PVs.TEC Configuration"=w331:T14)
            n173 = property class="Str"(reference=w336, "Value"="Selecting TEC Input...") -> ()  [unwired: 1 in, 2 out]
            n174 = call "meTEC_Set_ID 2000_Input Selection.vi"("Instance (1)"=u8 1, "error in (no error)"=w334, "TEC Configuration_IN"=w331, "Input Selection (ID 2000)"="meTEC_CH1_Input Selection (ID 2000)") -> ("error out"=w333:errorcluster)  [unwired: 5 in, 2 out]
          }
          frame "meTEC_CH1_Status (ID 2010)" {
            # "Aggiunto da Fede 27/04/2017\n\nObbiettivo: poter fare STATIC ON/OFF"
            n175 = Unbundle By Name(w342) -> ("PVs.TEC Configuration"=w340:T14)
            n176 = property class="Str"(reference=w344, "Value"="Selecting TEC Output stage...") -> ()  [unwired: 1 in, 2 out]
            n177 = call "meTEC_Set_ID 2010_Status.vi"("Instance (1)"=u8 1, "error in (no error)"=w339, "TEC Configuration_IN"=w340, "Status (ID 2010)"="meTEC_CH1_Status (ID 2010)") -> ("error out"=w338:errorcluster)  [unwired: 5 in, 2 out]
          }
          frame "meTEC_CH1_Object Target Temp. Source Selection (ID 50011)" {
            n178 = Unbundle By Name(w348) -> ("PVs.TEC Configuration"=w350:T14)
            n179 = property class="Str"(reference=w354, "Value"="Selecting TEC Object Target Temp. Source...") -> ()  [unwired: 1 in, 2 out]
            n180 = call "meTEC_Set_ID 50011_Object Target Temperature Source Selection.vi"("Instance (1)"=u8 1 ("Instance (0)"), "error in (no error)"=w352, "TEC Configuration_IN"=w350, "Object Target Temperature Source Selection (ID 50011)"="meTEC_CH1_Object Target Temp. Source Selection (ID 50011)") -> ("error out"=w351:errorcluster)  [unwired: 5 in, 2 out]
            n181 = Bundle By Name(cluster=w348, "PVs.Object Target Temperature Source_CH1"="meTEC_CH1_Object Target Temp. Source Selection (ID 50011)") -> (w347:T13)
            n182 = call "FGV_TE Controller.vi"("Operation (Read)"=FGV_Operations."Write", "FGV_TEC_IN"=w347) -> ()  [unwired: 8 in, 2 out]
          }
          frame "meTEC_CH1_Live Enable (ID 50000)" {
            n183 = Unbundle By Name(w358) -> ("PVs.TEC Configuration"=w357:T14)
            n184 = property class="Str"(reference=w362, "Value"="Enable / Disable Output...") -> ()  [unwired: 1 in, 2 out]
            n185 = call "meTEC_Set_ID 50000_Live Enable.vi"("Instance (1)"=u8 1 ("Instance (0)"), "error in (no error)"=w360, "TEC Configuration_IN"=w357, "Live Enable (ID 50000)"="meTEC_CH1_Live Enable (ID 50000)") -> ("error out"=w359:errorcluster)  [unwired: 5 in, 2 out]
          }
          frame "meTEC_CH1_Object Target Temperature (ID 3000 / 50012) [°C]" {
            # "0: ID 3000\n1: ID 50012"
            n186 = Unbundle By Name(w366) -> ("PVs.TEC Configuration"=w365:T14, "PVs.Object Target Temperature Source_CH1"=w363:u8)
            n187 = case shown="0, Default" w363 {
              tunnel: w369 -> [w376 w381]
              tunnel: [w375 w380] -> w368
              tunnel: "meTEC_CH1_Object Target Temperature (ID 3000 / 50012) [°C]" -> [w374 w379]
              tunnel: w365 -> [w373 w378]
              tunnel: u8 1 ("Instance") -> [w372 w377]
              frame 0, Default {
                n188 = call "meTEC_Set_ID 3000_Object Target Temperature.vi"("Instance (1)"=w372, "error in (no error)"=w376, "TEC Configuration_IN"=w373, "Object Target Temperature [°C]"=w374) -> ("error out"=w375:errorcluster)  [unwired: 5 in, 2 out]
              }
              frame 1 {
                n189 = call "meTEC_Set_ID 50012_Object Target Temperature.vi"("Instance (1)"=w377, "error in (no error)"=w381, "TEC Configuration_IN"=w378, "Object Target Temperature [°C]"=w379) -> ("error out"=w380:errorcluster)  [unwired: 5 in, 2 out]
              }
            }
            n190 = property class="Str"(reference=w371, "Value"="Setting TEC Object Target Temperature...") -> ()  [unwired: 1 in, 2 out]
          }
          frame "meTEC_CH1_Live Set Current (ID 50001) [A]" {
            n191 = Unbundle By Name(w385) -> ("PVs.TEC Configuration"=w384:T14)
            n192 = property class="Str"(reference=w389, "Value"="Setting TEC Live Set Current...") -> ()  [unwired: 1 in, 2 out]
            n193 = call "meTEC_Set_ID 50001_Live Set Current.vi"("Instance (1)"=u8 1 ("Instance"), "error in (no error)"=w387, "TEC Configuration_IN"=w384, "Live Current [A]"="meTEC_CH1_Live Set Current (ID 50001) [A]") -> ("error out"=w386:errorcluster)  [unwired: 5 in, 2 out]
          }
          frame "meTEC_CH1_Live Set Voltage (ID 50002) [V]" {
            n194 = Unbundle By Name(w393) -> ("PVs.TEC Configuration"=w392:T14)
            n195 = property class="Str"(reference=w397, "Value"="Setting TEC Live Set Voltage...") -> ()  [unwired: 1 in, 2 out]
            n196 = call "meTEC_Set_ID 50002_Live Set Voltage.vi"("Instance (1)"=u8 1 ("Instance"), "error in (no error)"=w395, "TEC Configuration_IN"=w392, "Live Set Voltage [V]"="meTEC_CH1_Live Set Voltage (ID 50002) [V]") -> ("error out"=w394:errorcluster)  [unwired: 5 in, 2 out]
          }
          frame "meTEC_Error Test 1_ID100_Device Type" {
            n197 = Unbundle By Name(w401) -> ("PVs.TEC Configuration"=w399:T14)
            n198 = property class="Str"(reference=w403, "Value"="Testing Error 1...") -> ()  [unwired: 1 in, 2 out]
            n199 = call "meTEC_Error Test_Read_ID 100_Device Type.vi"("error in (no error)"=w400, "TEC Configuration_IN"=w399) -> ("error out"=w398:errorcluster)  [unwired: 6 in, 3 out]
          }
          frame "meTEC_Perform Test" {
            # "Here you can place any VI for testing \nand execute it by pressing the \"Perform Test\" button\non the \"Error History\" tab."
            n200 = Unbundle By Name(w407) -> ("PVs.TEC Configuration"=w405:T14)
            n201 = property class="Str"(reference=w409, "Value"="Testing...") -> ()  [unwired: 1 in, 2 out]
            n202 = call "meTEC_Limit Read_ID 3000_Object Target Temperature.vi"("error in (no error)"=w406, "TEC Configuration_IN"=w405) -> ("error out"=w404:errorcluster)  [unwired: 6 in, 3 out]
          }
        }
      }
      frame " ----- Arduino Functions ----- " {
      }
      frame "Read Arduino Serial" {
        n203 = global read "Global_Initialized.vi" "Initialized_Step_Arduino?"() -> (w411:bool)
        n204 = case shown="True" w411 {
          tunnel: w414 -> [_ _]
          tunnel: [w415 w422] -> w410
          tunnel: w412 -> [_ w428]
          tunnel: w413 -> [w415 _]
          frame False {
          }
          frame True {
            n205 = call "FGV_TE Controller.vi"() -> ("error out"=w420:errorcluster, "FGV_TEC_OUT"=w421:T13)  [unwired: 10 in]
            n206 = Unbundle By Name(w421) -> ("Arduino VISA"=w425:refnum<visa-resource-name>)
            n207 = property class="Str"(reference=w428) -> (reference out=w431:refnum<vi>, "Value"=w426:string)  [unwired: 1 in, 1 out]
            n208 = call "serial_read.vi"("error in (no error)"=w420, "VISA Refnum in"=w425) -> ("error out"=w424:errorcluster, "read buffer"=w423:string)  [unwired: 8 in]
            n209 = Concatenate Strings(w426, w423) -> (w416:string)
            n210 = property class="Str"(reference=w431, error in=w424, "Value"=w416) -> (reference out=w429:refnum<vi>, error out=w427:errorcluster)
            n211 = String Length(string=w416) -> (length=w418:i32)
            n212 = Greater Or Equal?(x=w418, y=41) -> (x >= y?=w417:bool)
            n213 = case shown="True" w417 {
              tunnel: [w432 w454] -> w430
              tunnel: w416 -> [w432 w453]
              frame False {
              }
              frame True {
                # "Aggiungere if se c'è errore"
                n214 = call "tec_global_data_typedef.vi"() -> ("Numeric Control 2"=w445:T1)  [unwired: 11 in]
                n215 = call "packet_elaborate.vi"("String in"=w453) -> ("Numeric Control"=w446:T19, "String out"=w454:string)  [unwired: 9 in]
                n216 = Unbundle By Name(w446) -> ("Data"=w451:i64[])  [unwired: 1 out]
                n217 = Unbundle By Name(w446) -> ("Type"=w444:string, "Sequence"=w442:u16, "Data"=w441:i64[], "CS"=w440:u16, "CRC"=w439:u16, "Time Stamp"=w438:timestamp)
                n218 = Unbundle By Name(w445) -> ("Voltage"=w437:dbl, "Current"=w436:dbl, "SinkT"=w435:dbl, "ObjT"=w434:dbl)  [unwired: 1 out]
                n219 = Index Array(array=w451, index #1=0 ("index"), index #2=1 ("index")) -> (element #1=→"Monitor Chart_ARD 1" →"ARD_ Object Temperature [°C] 1":i64, element #2=→"Monitor Chart_ARD 2" →"ARD_Object Temperature [°C] 2":i64)
                n220 = Bundle By Name(cluster=T19 {"Type"="", "Sequence"=0, "Data"=[], "CS"=0, "CRC"=0, "Time Stamp"=timestamp(0 s since 1904-01-01), "Voltage"=0.0, "Current"=0.0, "TEC T_1"=0.0, "TEC T_2"=0.0} ("Numeric Control"), "Type"=w444, "Sequence"=w442, "Data"=w441, "CS"=w440, "CRC"=w439, "Time Stamp"=w438, "Voltage"=w437, "Current"=w436, "TEC T_1"=w435, "TEC T_2"=w434) -> (w433:T19)
                n221 = call "global_data.vi"("Operation (Read)"=FGV_Operations."Write", "Numeric Control"=w433) -> ()  [unwired: 9 in, 1 out]
              }
            }
            n222 = property class="Str"(reference=w429, error in=w427, "Value"=w430) -> (error out=w422:errorcluster)  [unwired: 1 out]
          }
        }
      }
      frame "Disconnect Arduino" {
        n223 = call "FGV_TE Controller.vi"() -> ("error out"=w456:errorcluster, "FGV_TEC_OUT"=w459:T13)  [unwired: 10 in]
        n224 = Unbundle By Name(w459) -> ("Arduino VISA"=w458:refnum<visa-resource-name>)
        n225 = VISA Clear(VISA resource name=w458, error in (no error)=w456) -> (VISA resource name out=w457:refnum<visa-resource-name>, error out=w455:errorcluster)
        n226 = VISA Close(VISA resource name=w457, error in (no error)=w455) -> ()  [unwired: 1 out]
      }
      frame "  -----  File manager  ----- " {
      }
      frame "Add recording" {
        w465 = T20 {"Start"=timestamp(0 s since 1904-01-01), "Finish"=timestamp(0 s since 1904-01-01), "Duration"=0}  # record session
        n227 = Multiply(x="Duration (minutes)", y=60) -> (x*y=w463:i32)
        n228 = Add(x="Recording start time", y=w463) -> (x+y=w464:timestamp)
        n229 = Bundle By Name(cluster=w465, "Start"="Recording start time", "Finish"=w464, "Duration"="Duration (minutes)") -> (w466:T20)
        n230 = call "record_sessions.vi"("Operation (Read)"=FGV_Operations."Write", "record session"=w466) -> ()  [unwired: 8 in, 2 out]
      }
      frame "Update table" {
        n231 = call "record_sessions.vi"() -> ("record sessions"=w469:T20[])  [unwired: 10 in, 1 out]
        n232 = for {
          tunnel: w469 -> [w475] mode=indexing
          tunnel: [w476] -> w468 mode=indexing
          n233 = Unbundle By Name(w475) -> ("Start"=w474:timestamp, "Finish"=w470:timestamp, "Duration"=w473:i32)
          n234 = Format Date/Time String(seconds (now)=w474) -> (date/time string=w477:string)  [unwired: 2 in]
          n235 = Format Date/Time String(seconds (now)=w470) -> (date/time string=w471:string)  [unwired: 2 in]
          n236 = Number To Decimal String(number=w473) -> (decimal integer string=w472:string)  [unwired: 1 in]
          n237 = Build Array(w477, w471, w472) -> (w476:string[])
        }
        n238 = property on="Planned Recordings" class="MCListbox (strict)"("ItemNames"=w468) -> ()  [unwired: 2 in, 2 out]
      }
      frame "Start new recording" {
        n239 = control-ref of="Reference timestamp 2"() -> (w478:refnum<vi>)
        n240 = control-ref of="TEC Log File"() -> (w479:refnum<vi>)
        n241 = call "start_new_recording.vi"("error in (no error)"=w481, "reference in"=w478, "Path in"=w479) -> ("error out"=w480:errorcluster)  [unwired: 8 in]
      }
      frame "Save to log file" {
        n242 = global read "Global_Initialized.vi" "Initialized_Step_Arduino?"() -> (w483:bool)
        n243 = case shown="True" w483 {
          tunnel: [_ w484] -> w482
          frame False {
          }
          frame True {
            n244 = call "FGV_TE Controller.vi"() -> ("error out"=w485:errorcluster, "FGV_TEC_OUT"=w489:T13)  [unwired: 10 in]
            n245 = Unbundle By Name(w489) -> ("TEC Log File"=w486:path)
            n246 = call "global_data.vi"("Operation (Read)"=FGV_Operations."Read and delete") -> ("Array"=w487:T19[])  [unwired: 10 in]
            n247 = for {
              N -> [w495]
              tunnel: w487 -> [w493] mode=indexing
              tunnel: w486 -> [w498]
              shift-right: [w490] -> w484
              shift-left: w485 -> [w491]
              i -> [w497]
              n248 = local read "Reference timestamp 2"() -> (w492:timestamp)
              n249 = Decrement(x=w495) -> (x-1=w494:i32)
              n250 = Equal?(x=w494, y=w497) -> (x = y?=w496:bool)
              n251 = call "file_log_save.vi"("Reference timestamp"=w492, "error in (no error)"=w491, "Flush?"=w496, "Numeric Control"=w493, "TEC Log File"=w498) -> ("error out"=w490:errorcluster)  [unwired: 6 in]
            }
          }
        }
      }
    }
  }
  n252 = while "Event Handling Loop" {
    tunnel: w1 -> [w501]
    tunnel: w16 -> [w500]
    stop <- w502 stop-if-true
    # ">> Error Queue >>"
    # ">> Main Queue >>"
    n253 = event shown="[12] \"Reconnect Arduino\": Value Change" {
      selector: _ -> [_ _ _ _ _ _ _ _ _ _ _ _ _ _ _ _ _ _ _]
      dyn-events: _ -> [_ _ _ _ _ _ _ _ _ _ _ _ _ _ _ _ _ _ _]
      timeout: _ -> [_ _ _ _ _ _ _ _ _ _ _ _ _ _ _ _ _ _ _]
      tunnel: [w510 w515 w522 w525 w531 w537 w543 w549 w555 w561 w567 w573 w578 w582 w588 w590 w595 w601 w607] -> w503
      tunnel: [w505 _ w517 _ _ _ _ _ _ _ _ _ _ _ _ _ _ _ _] -> w502
      tunnel: [errorcluster {"status"=FALSE, "code"=5000, "source"=""} ("element") _ errorcluster {"status"=FALSE, "code"=5000, "source"=""} ("element") _ _ _ _ _ _ _ _ _ _ _ _ _ _ _ _] -> w499
      event Application Instance Close? {
        n254 = event-data() -> ()  [unwired: 1 in, 4 out]
        n255 = Two Button Dialog(message="Are you sure you want to quit?") -> (T button?=w505:bool)  [unwired: 2 in]
        n256 = Select(t=T10[] [{"Parameter"="", "Variant"=variant, "Main Loop States"=enum."Shutdown"}] ("Elements to enqueue (Array)"), s=w505, f=T10[] [{"Parameter"="", "Variant"=variant, "Main Loop States"=enum."Idle"}] ("Elements to enqueue (Array)")) -> (s? t:f=w510:T10[])
        n257 = global write "Global_Quit.vi" "Quit"(w505) -> ()
        n258 = event-data("Discard?"=TRUE) -> ()  [unwired: 2 in, 1 out]
      }
      event "Add recording": Value Change {
        n259 = event-data() -> ()  [unwired: 1 in, 6 out]
        n260 = local write "Add recording"(FALSE ("Add Recording")) -> ()
        n261 = Build Array(T10 {"Parameter"="", "Variant"=variant, "Main Loop States"=enum."Add recording"} ("Main Loop Queue Data"), T10 {"Parameter"="", "Variant"=variant, "Main Loop States"=enum."Update table"} ("Main Loop Queue Data"), T10 {"Parameter"="", "Variant"=variant, "Main Loop States"=enum."Idle"} ("Main Loop Queue Data")) -> (w515:T10[])
      }
      event Panel Close? {
        n262 = event-data() -> ()  [unwired: 1 in, 3 out]
        n263 = Two Button Dialog(message="Are you sure you want to quit?") -> (T button?=w517:bool)  [unwired: 2 in]
        n264 = Select(t=T10[] [{"Parameter"="", "Variant"=variant, "Main Loop States"=enum."Shutdown"}] ("Elements to enqueue (Array)"), s=w517, f=T10[] [{"Parameter"="", "Variant"=variant, "Main Loop States"=enum."Idle"}] ("Elements to enqueue (Array)")) -> (s? t:f=w522:T10[])
        n265 = global write "Global_Quit.vi" "Quit"(w517) -> ()
        n266 = event-data("Discard?"=TRUE) -> ()  [unwired: 1 in, 1 out]
      }
      event Value Change {
        n267 = event-data() -> ("CtlRef"=w524:refnum<vi>)  [unwired: 1 in, 4 out]
        n268 = property class="Ring (strict)"(reference=w524) -> ("Label.Text"=w527:string)  [unwired: 1 in, 2 out]
        n269 = Bundle By Name(cluster=T10 {"Parameter"="", "Variant"=variant, "Main Loop States"=enum."TE Controller"} ("Main Loop Queue Data"), "Parameter"=w527) -> (w526:T10)
        n270 = Build Array(w526, T10 {"Parameter"="", "Variant"=variant, "Main Loop States"=enum."Idle"} ("Main Loop Queue Data")) -> (w525:T10[])
      }
      event Value Change {
        n271 = event-data() -> ("CtlRef"=w530:refnum<vi>)  [unwired: 1 in, 4 out]
        n272 = property class="Ring (strict)"(reference=w530) -> ("Label.Text"=w533:string)  [unwired: 1 in, 2 out]
        n273 = Bundle By Name(cluster=T10 {"Parameter"="", "Variant"=variant, "Main Loop States"=enum."TE Controller"} ("Main Loop Queue Data"), "Parameter"=w533) -> (w532:T10)
        n274 = Build Array(w532, T10 {"Parameter"="", "Variant"=variant, "Main Loop States"=enum."Idle"} ("Main Loop Queue Data")) -> (w531:T10[])
      }
      event Value Change {
        n275 = event-data() -> ("CtlRef"=w536:refnum<vi>)  [unwired: 1 in, 4 out]
        n276 = property class="Ring (strict)"(reference=w536) -> ("Label.Text"=w539:string)  [unwired: 1 in, 2 out]
        n277 = Bundle By Name(cluster=T10 {"Parameter"="", "Variant"=variant, "Main Loop States"=enum."TE Controller"} ("Main Loop Queue Data"), "Parameter"=w539) -> (w538:T10)
        n278 = Build Array(w538, T10 {"Parameter"="", "Variant"=variant, "Main Loop States"=enum."Idle"} ("Main Loop Queue Data")) -> (w537:T10[])
      }
      event Value Change {
        n279 = event-data() -> ("CtlRef"=w541:refnum<vi>)  [unwired: 1 in, 5 out]
        n280 = property class="Ring (strict)"(reference=w541) -> ("Label.Text"=w545:string)  [unwired: 1 in, 2 out]
        n281 = Bundle By Name(cluster=T10 {"Parameter"="", "Variant"=variant, "Main Loop States"=enum."TE Controller"} ("Main Loop Queue Data"), "Parameter"=w545) -> (w544:T10)
        n282 = Build Array(w544, T10 {"Parameter"="", "Variant"=variant, "Main Loop States"=enum."Idle"} ("Main Loop Queue Data")) -> (w543:T10[])
      }
      event "meTEC_CH1_Object Target Temperature (ID 3000 / 50012) [°C]": Value Change {
        n283 = event-data() -> ("CtlRef"=w548:refnum<vi>)  [unwired: 1 in, 4 out]
        n284 = property class="DigNum (strict)"(reference=w548) -> ("Label.Text"=w551:string)  [unwired: 1 in, 2 out]
        n285 = Bundle By Name(cluster=T10 {"Parameter"="", "Variant"=variant, "Main Loop States"=enum."TE Controller"} ("Main Loop Queue Data"), "Parameter"=w551) -> (w550:T10)
        n286 = Build Array(w550, T10 {"Parameter"="", "Variant"=variant, "Main Loop States"=enum."Idle"} ("Main Loop Queue Data")) -> (w549:T10[])
      }
      event "meTEC_CH1_Live Set Current (ID 50001) [A]": Value Change {
        n287 = event-data() -> ("CtlRef"=w554:refnum<vi>)  [unwired: 1 in, 4 out]
        n288 = property class="DigNum (strict)"(reference=w554) -> ("Label.Text"=w557:string)  [unwired: 1 in, 2 out]
        n289 = Bundle By Name(cluster=T10 {"Parameter"="", "Variant"=variant, "Main Loop States"=enum."TE Controller"} ("Main Loop Queue Data"), "Parameter"=w557) -> (w556:T10)
        n290 = Build Array(w556, T10 {"Parameter"="", "Variant"=variant, "Main Loop States"=enum."Idle"} ("Main Loop Queue Data")) -> (w555:T10[])
      }
      event "meTEC_CH1_Live Set Voltage (ID 50002) [V]": Value Change {
        n291 = event-data() -> ("CtlRef"=w560:refnum<vi>)  [unwired: 1 in, 4 out]
        n292 = property class="DigNum (strict)"(reference=w560) -> ("Label.Text"=w563:string)  [unwired: 1 in, 2 out]
        n293 = Bundle By Name(cluster=T10 {"Parameter"="", "Variant"=variant, "Main Loop States"=enum."TE Controller"} ("Main Loop Queue Data"), "Parameter"=w563) -> (w562:T10)
        n294 = Build Array(w562, T10 {"Parameter"="", "Variant"=variant, "Main Loop States"=enum."Idle"} ("Main Loop Queue Data")) -> (w561:T10[])
      }
      event "meTEC_Reset Device": Value Change {
        n295 = event-data() -> ("CtlRef"=w566:refnum<vi>)  [unwired: 1 in, 4 out]
        n296 = property class="Bool"(reference=w566) -> ("Label.Text"=w569:string)  [unwired: 1 in, 2 out]
        n297 = Bundle By Name(cluster=T10 {"Parameter"="", "Variant"=variant, "Main Loop States"=enum."TE Controller"} ("Main Loop Queue Data"), "Parameter"=w569) -> (w568:T10)
        n298 = Build Array(w568, T10 {"Parameter"="Return Front Panel Controls to TEC Reset State", "Variant"=variant, "Main Loop States"=enum."TE Controller"} ("Main Loop Queue Data")) -> (w567:T10[])
      }
      event "meTEC_Reset Device 2": Value Change {
        n299 = event-data() -> ("CtlRef"=w572:refnum<vi>)  [unwired: 1 in, 4 out]
        n300 = property class="Bool"(reference=w572) -> ("Label.Text"=w575:string)  [unwired: 1 in, 2 out]
        n301 = Bundle By Name(cluster=T10 {"Parameter"="", "Variant"=variant, "Main Loop States"=enum."TE Controller"} ("Main Loop Queue Data"), "Parameter"=w575) -> (w574:T10)
        n302 = Build Array(w574, T10 {"Parameter"="Return Front Panel Controls to TEC Reset State", "Variant"=variant, "Main Loop States"=enum."TE Controller"} ("Main Loop Queue Data")) -> (w573:T10[])
      }
      event "Reconnect Arduino": Value Change {
        n303 = event-data() -> ()  [unwired: 1 in, 6 out]
        n304 = local write "Reconnect Arduino"(FALSE ("Reconnect Arduino")) -> ()
        n305 = Build Array(T10 {"Parameter"="", "Variant"=variant, "Main Loop States"=enum."Initialize Arduino"} ("Main Loop Queue Data"), T10 {"Parameter"="", "Variant"=variant, "Main Loop States"=enum."Idle"} ("Main Loop Queue Data")) -> (w578:T10[])
      }
      event "Reconnect Tec": Value Change {
        n306 = event-data() -> ()  [unwired: 1 in, 6 out]
        n307 = local write "Reconnect Tec"(FALSE ("Reconnect Tec")) -> ()
        n308 = Build Array(T10 {"Parameter"="", "Variant"=variant, "Main Loop States"=enum."Initialize"} ("Main Loop Queue Data"), T10 {"Parameter"="", "Variant"=variant, "Main Loop States"=enum."Idle"} ("Main Loop Queue Data")) -> (w582:T10[])
      }
      event "meTEC_Initialize Device": Value Change {
        # "Reset boolean control to\ninitial value"
        n309 = event-data() -> ()  [unwired: 1 in, 1 out]
        n310 = local write "meTEC_Initialize Device"(FALSE ("meTEC_Initialize Device")) -> ()
        n311 = Build Array(T10 {"Parameter"="", "Variant"=variant, "Main Loop States"=enum."Initialize"} ("Main Loop Queue Data"), T10 {"Parameter"="", "Variant"=variant, "Main Loop States"=enum."Idle"} ("Main Loop Queue Data")) -> (w588:T10[])
      }
      event "save log file": Value Change {
        n312 = event-data() -> ()  [unwired: 1 in, 6 out]
        n313 = local write "save log file"(FALSE ("save log file")) -> ()
        n314 = Build Array(T10 {"Parameter"="", "Variant"=variant, "Main Loop States"=enum."Save to log file"} ("Main Loop Queue Data"), T10 {"Parameter"="", "Variant"=variant, "Main Loop States"=enum."Idle"} ("Main Loop Queue Data")) -> (w590:T10[])
        n315 = One Button Dialog(message="sffdvc") -> ()  [unwired: 1 in, 1 out]
      }
      event "Read Arduino Serial": Value Change {
        n316 = event-data() -> ()  [unwired: 1 in, 6 out]
        n317 = local write "Read Arduino Serial"(FALSE ("Read Arduino Serial")) -> ()
        n318 = Build Array(T10 {"Parameter"="", "Variant"=variant, "Main Loop States"=enum."Read Arduino Serial"} ("Main Loop Queue Data"), T10 {"Parameter"="", "Variant"=variant, "Main Loop States"=enum."Idle"} ("Main Loop Queue Data")) -> (w595:T10[])
        n319 = One Button Dialog(message="sffdvc") -> ()  [unwired: 1 in, 1 out]
      }
      event "meTEC_Error Test 1_ID100_Device Type": Value Change {
        n320 = event-data() -> ("CtlRef"=w600:refnum<vi>)  [unwired: 1 in, 4 out]
        n321 = property class="Bool"(reference=w600) -> ("Label.Text"=w603:string)  [unwired: 1 in, 2 out]
        n322 = Bundle By Name(cluster=T10 {"Parameter"="", "Variant"=variant, "Main Loop States"=enum."TE Controller"} ("Main Loop Queue Data"), "Parameter"=w603) -> (w602:T10)
        n323 = Build Array(w602, T10 {"Parameter"="", "Variant"=variant, "Main Loop States"=enum."Idle"} ("Main Loop Queue Data")) -> (w601:T10[])
      }
      event "meTEC_Perform Test": Value Change {
        n324 = event-data() -> ("CtlRef"=w606:refnum<vi>)  [unwired: 1 in, 4 out]
        n325 = property class="Bool"(reference=w606) -> ("Label.Text"=w609:string)  [unwired: 1 in, 2 out]
        n326 = Bundle By Name(cluster=T10 {"Parameter"="", "Variant"=variant, "Main Loop States"=enum."TE Controller"} ("Main Loop Queue Data"), "Parameter"=w609) -> (w608:T10)
        n327 = Build Array(w608, T10 {"Parameter"="", "Variant"=variant, "Main Loop States"=enum."Idle"} ("Main Loop Queue Data")) -> (w607:T10[])
      }
    }
    n328 = call "Multiple Element Enqueue - Main Loop.vi"("Elements to enqueue (Array)"=w503, "Queue In"=w501) -> ()  [unwired: 8 in, 2 out]
    n329 = call "Error Queue - Enqueue Element.vi"("error in (no error)"=w499, "Error Queue IN"=w500) -> ()  [unwired: 9 in, 1 out]
  }
  n330 = timed-loop {
    tunnel: w1 -> [w612]
    timing: w7 -> [_]
    timing-out: [_] -> w6
    stop <- w613 stop-if-true
    # "Save log file routine"
    n331 = node-c288() -> ()  [unwired: 1 in, 1 out]
    n332 = global read "Global_Initialized.vi" "Initialized_Step_Arduino?"() -> (w611:bool)
    "Arduino Connected" <- w611
    n333 = case shown="True" w611 {
      tunnel: w612 -> [_ w617]
      frame False {
      }
      frame True {
        n334 = Build Array(T10 {"Parameter"="", "Variant"=variant, "Main Loop States"=enum."Read Arduino Serial"} ("Main Loop Queue Data"), T10 {"Parameter"="", "Variant"=variant, "Main Loop States"=enum."Idle"} ("Main Loop Queue Data")) -> (w614:T10[])
        n335 = call "Multiple Element Enqueue - Main Loop.vi"("Elements to enqueue (Array)"=w614, "Queue In"=w617) -> ()  [unwired: 8 in, 2 out]
      }
    }
    n336 = global read "Global_Quit.vi" "Quit"() -> (w613:bool)
    n337 = node-c288() -> ()  [unwired: 1 in, 1 out]
  }
  n338 = timed-loop {
    tunnel: w1 -> [w621]
    timing: w11 -> [_]
    timing-out: [_] -> w10
    stop <- w620 stop-if-true
    # "Save log file routine"
    n339 = node-c288() -> ()  [unwired: 1 in, 1 out]
    n340 = Build Array(T10 {"Parameter"="", "Variant"=variant, "Main Loop States"=enum."Save to log file"} ("Main Loop Queue Data"), T10 {"Parameter"="", "Variant"=variant, "Main Loop States"=enum."Idle"} ("Main Loop Queue Data")) -> (w622:T10[])
    n341 = call "Multiple Element Enqueue - Main Loop.vi"("Elements to enqueue (Array)"=w622, "Queue In"=w621) -> ()  [unwired: 8 in, 2 out]
    n342 = global read "Global_Quit.vi" "Quit"() -> (w620:bool)
    n343 = node-c288() -> ()  [unwired: 1 in, 1 out]
  }
  n344 = timed-loop {
    tunnel: w1 -> [w628]
    timing: w4 -> [_]
    timing-out: [_] -> w3
    stop <- w629 stop-if-true
    # "Save log file routine"
    n345 = node-c288() -> ()  [unwired: 1 in, 1 out]
    n346 = global read "Global_Initialized.vi" "Initialized_Step_Arduino?"() -> (w627:bool)
    n347 = case shown="True" w627 {
      tunnel: w628 -> [_ w630]
      frame False {
      }
      frame True {
        n348 = call "new_rec.vi"("Queue in"=w630) -> ()  [unwired: 11 in]
      }
    }
    n349 = global read "Global_Quit.vi" "Quit"() -> (w629:bool)
    n350 = node-c288() -> ()  [unwired: 1 in, 1 out]
  }
  n351 = node-c288(w6) -> ()  [unwired: 1 out]
  n352 = node-c288(w10) -> ()  [unwired: 1 out]
  n353 = node-c288(w3) -> ()  [unwired: 1 out]
  n354 = Merge Errors(w8, w34, w17) -> (w33:errorcluster)
  n355 = call <vilib>:"General Error Handler.vi"("error in (no error)"=w33) -> ("error out"=w28:errorcluster)  [unwired: 10 in, 4 out]
  n356 = call "Clear All Errors.vi"("error in (no error)"=w28) -> ("error out"=w23:errorcluster)  [unwired: 1 in]
  n357 = property class="App"(error in=w23) -> ("App.Kind"=w40:T11)  [unwired: 1 in, 2 out]
  n358 = Equal?(x=w40, y=T11."Run Time System") -> (x = y?=w38:bool)
  n359 = Quit LabVIEW(quit? (T)=w38) -> ()
